vi "UI.vi"(0 "reference in":refnum<class "GUI Data Viewer.lvclass">, 5 "error in (no error)":errorcluster) -> (14 "reference out":refnum<class "GUI Data Viewer.lvclass">, 19 "error out":errorcluster)   [LabVIEW 2019, in "GUI Data Viewer.lvclass"]
uses:
  GUI Data Viewer.lvclass
  D:/GIT H4000/H4000/src/GUI_class/GUI.lvclass
  TypeDef/GUI Data Motor.ctl
  TypeDef/State Engine.ctl
  TypeDef/Needle Valve State.ctl
  GUI_class/GUI.lvclass/GUI.ctl
  TypeDef/AI_Data_Array.ctl
  TypeDef/AI_Data.ctl
  TypeDef/AI Statistics Data.ctl
  TypeDef/CalibrationData.ctl
  TypeDef/GUI Setting Channel.ctl
  TypeDef/GUI AI Ranges.ctl
  TypeDef/Scale Data.ctl
  SV_Wrap/SharedVariableWrapper.lvclass/SharedVariableWrapper.ctl
  TypeDef/Data Stand.ctl
  TypeDef/Mode.ctl
  TypeDef/ExecuteStepState.ctl
  TypeDef/Direction.ctl
  Modbus_class/STS REG.ctl
  TypeDef/SP_TYPE.ctl
  TypeDef/State 44-1-2.ctl
  Logger_class/Current Alarms.ctl
  Logger_class/EventData.ctl
  TypeDef/AlarmType.ctl
  TypeDef/error.ctl
  TypeDef/TCP Connection List.ctl
  <vilib>/NI/Modbus Library/Network Protocol/Network Slave/TCP/Connection.ctl
  TypeDef/Needle Valve Data.ctl
  modbus engine custom/MB_ENGINE_class/Engine State.ctl
  modbus engine custom/MB_ENGINE_class/Engine Alarms.ctl
  modbus engine custom/MB_ENGINE_class/Settings.ctl
  modbus engine custom/MB_ENGINE_class/Limits Status.ctl
  TypeDef/State PMG.ctl
  TypeDef/PMG Mode.ctl
  TypeDef/State Engine 2.ctl
  Modbus_class/CMD REG.ctl
  MessageAMC_class/MessageAMC.lvclass
  D:/GIT H4000/H4000/src/MessageInterface_class/MessageInterface.lvclass
  dd5645e7-7e6e-4691-95a0-f3999e380403.vi
  7c45c07e-402c-4694-b421-37bbb0792970.vi
  9a17e93e-f953-4ee5-a306-57728009cce8.vi
  49e40455-3b35-4e41-8043-7be2530b05e7.vi
  18541d12-0d59-4aa6-b87b-abaa8bd8a6e4.vi
  0b4675b1-6847-4ac1-af90-c3adb7e73b02.vi
  a37d2d01-2c81-48ed-b054-fbf1630c5e7f.vi
  1656e42f-8660-4372-8b8f-7d4878a983bb.vi
  0bfe0e00-7643-4872-b052-8b7f26ea950b.vi
  ffb61635-9317-4c26-9d6e-9a19723cfb80.vi
  07359d59-ff70-46be-ab7b-6b377f7d411b.vi
  f6869450-7c10-4810-a35a-46c2f9ab3114.vi
  d18fabfa-1a79-49d4-a75c-348c28269d79.vi
  d5087eaa-c132-4133-aa21-01cfea8cde9e.vi
  bf1f9f25-528c-4176-8d10-e7cb21e5fec2.vi
  e75bdee8-ee2a-4a87-80aa-f3e942366e41.vi
  f0a45f4a-50aa-43d2-a935-47ced4280b1d.vi
  cedc6c5e-9abe-42eb-b0bd-72af6e3c241b.vi
  GUI_class/Set Win State.vi
  GUI_class/protected/GetSheredData.vi
  dd5645e7-7e6e-4691-95a0-f3999e380403.vi/b5fe87cb-a842-48a6-ac33-23eb568e7aa4.vi
  SV_Wrap/Write Var Info.vi
  SV_Wrap/Read Var Info.vi
  7c45c07e-402c-4694-b421-37bbb0792970.vi/dcc16439-89b0-4283-9d30-44b050a4d697.vi
  49e40455-3b35-4e41-8043-7be2530b05e7.vi/daf86f20-c8fb-4d87-9d07-c45676e1c3eb.vi
  0b4675b1-6847-4ac1-af90-c3adb7e73b02.vi/1200fe38-aa22-4cab-916d-93cea7720ab1.vi
  a37d2d01-2c81-48ed-b054-fbf1630c5e7f.vi/408f54e3-e009-4e36-949a-cd8d2e669441.vi
  1656e42f-8660-4372-8b8f-7d4878a983bb.vi/3922be2e-8b70-4363-9278-b2eb396c106a.vi
  0bfe0e00-7643-4872-b052-8b7f26ea950b.vi/6182aae4-c240-425b-9f2c-7ffeca9a8282.vi
  07359d59-ff70-46be-ab7b-6b377f7d411b.vi/4407c637-9fa4-4312-8a7e-15880992c60d.vi
  f6869450-7c10-4810-a35a-46c2f9ab3114.vi/792ba656-e40c-479d-9018-d5581bd1c278.vi
  d18fabfa-1a79-49d4-a75c-348c28269d79.vi/30a4da04-0b22-486b-9a8e-f683f1398578.vi
  bf1f9f25-528c-4176-8d10-e7cb21e5fec2.vi/3b2418f1-7f16-47c7-ba27-2bc06ef6e628.vi
  e75bdee8-ee2a-4a87-80aa-f3e942366e41.vi/2202224e-9635-4547-b368-63a478ce0b2e.vi
  f0a45f4a-50aa-43d2-a935-47ced4280b1d.vi/85cd7a43-9f39-4f72-add9-b75505d0e5f9.vi
  cedc6c5e-9abe-42eb-b0bd-72af6e3c241b.vi/f9761a82-5467-46da-8b92-b56c6279bfed.vi
  SV_Wrap/Read connection str.vi
  <userlib>/_OpenG.lib/time/time.llb/Tick Count (ms)__ogtk.vi
  GUI_class/GUI.lvclass
  MessageInterface_class/MessageInterface.lvclass
  SV_Wrap/SharedVariableWrapper.lvclass
  modbus engine custom/MB_ENGINE_class/MB_ENGINE.lvclass
  <vilib>/NI/Modbus Library/Network Protocol/Network Slave/TCP/TCP Slave.lvclass
panel:
  out "chmbr 2":dbl(graph) caption="41.3 [МПа]"
  out "leak":dbl caption="Утечки [МПа/мин]" format="%.2f"
  out "modbus":bool caption="Модбас"
  out "size(s) 2":i32 caption="Кол-во активных"
  out "size(s)":i32 caption="Общее кол-во"
  out "Active":string[](array[string]) caption="Активные подключения"
  out "База данных":bool
  out "warning":bool caption="Предупреждение"
  out "alarm":bool caption="Авария"
  out "String":string
  in  "Tab Control":enum32{"Аварии / предупреждения", "Графики"}(tab)
  out "Multicolumn Listbox":i32(listbox)=-1
  in  "Clear Error":bool
  out "dut":T1(graph) caption="Образец [МПа]"
  out "chmbr":T1(graph) caption="Камера [МПа]"
  in  "remote":bool caption="Разрешить внешнее управление"
  out "P_DUT_MB":dbl caption="Образец  [МПа]" format="%.2f"
  out "P_CHMBR_MB":dbl caption="Камера [МПа]" format="%.2f"
  out "Angle 37 2":dbl caption="Угол, град" format="%#.1f град"
  out "StateValveModbus 2":T2
  out "StateValveModbus":T2
  in  "alarm press":bool
  out "Angle 37 1":dbl caption="Угол, град" format="%#.1f град"
  out "m24":T3
  out "m21":T3
  out "m12":T3
  out "AO 1":dbl caption="Напр. проп. клапан [В]" format="%.2f"
  out "AO 0":dbl caption="Напр.\nпроп.\nклапан [В]" format="%.2f"
  out "30":dbl(slide)=60.30534351145039 caption="НВД" scale=0.0..10.0
  in  "stop":bool
  out "Connect":bool caption="Подключение \nконтроллер"
  out "DO 7":bool caption="33.9"
  out "DO 6":bool caption="33.8"
  out "DO 11":bool caption="33.13"
  out "DO 8":bool caption="33.12"
  out "5.1":dbl(slide)=60.30534351145039 scale=0.0..100.0
  out "4.1":dbl(slide)=53.84615384615385 scale=0.0..100.0
  out "5.2":dbl(slide)=60.30534351145039 scale=0.0..100.0
  out "4.2":dbl(slide)=53.84615384615385 scale=0.0..100.0
  out "41.2 [МПа]":dbl(knob) scale=0.0..10.0
  out "41.1 [МПа]":dbl(knob) scale=0.0..10.0
  out "38.3 [МПа]":dbl(knob) scale=0.0..10.0
  out "38.2 [МПа]":dbl(knob) scale=0.0..10.0
  out "41.3 [МПа]":dbl(knob) scale=0.0..10.0
  out "38.1 [МПа]":dbl(knob) scale=0.0..500.0
  out "DO 18":bool caption="ВОЗДУХ"
  out "44.1":bool
  out "44.2":bool
  out "37.2":bool
  out "37.1":bool
  out "DO 14":bool caption="33.6"
  out "DO 16":bool caption="33.4"
  out "DO 15":bool caption="33.5"
  out "DO 13":bool caption="33.10"
  out "DO 12":bool caption="33.11"
  out "DO 17":bool caption="33.3"
  out "DO 10":bool caption="33.2"
  out "DO 9":bool caption="33.1"
  out "DO 5":bool caption="33.7"
  out "nitro":bool
  # "42  бюретка"
  # "Подключения модбас"
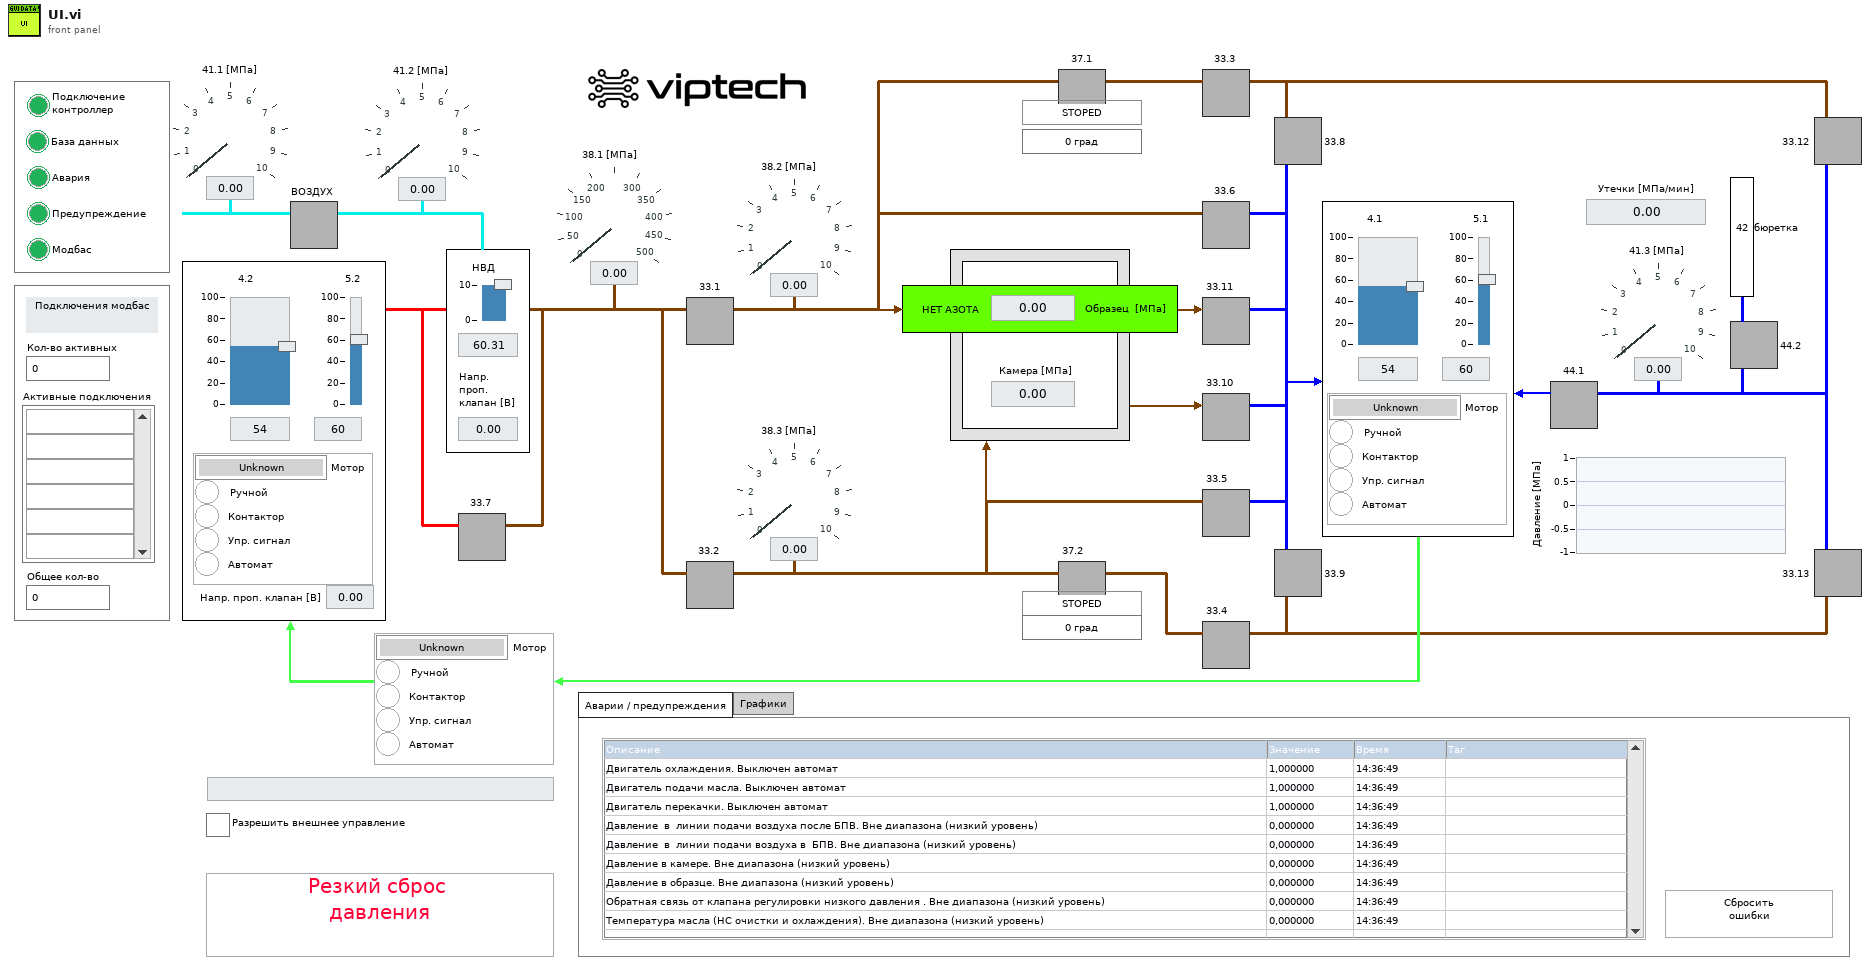
[diagram p1: front panel]
types:
  T1 = cluster{"Pressure SP":dbl, "scl mean 1Hz":dbl, "scl mean 1Hz":dbl}
  T2 = typedef "Needle Valve State.ctl" = enum16{"STOPED", "CLOSED", "OPENED", "OPENING", "CLOSING", "FULL_CLOSE"}
  T3 = typedef "GUI Data Motor.ctl" = cluster{"EngState":T4, "Active":bool, "Contactor":bool, "CMD":bool, "Automat":bool}
  T4 = typedef "State Engine.ctl" = enum16{"Unknown", "Off", "TupningOn", "On", "TurningOff"}
  T5 = typedef "CalibrationData.ctl" = cluster{"Channels":T6[], "Scales":T8[]}
  T6 = typedef "GUI Setting Channel.ctl" = cluster{"Name":string, "AI Ranges":T7, "ScaleIndex":u32}
  T7 = typedef "GUI AI Ranges.ctl" = cluster{"HI":bool, "HIHI":bool, "LO":bool, "LOLO":bool, "HIHI VAL":dbl, "HI VAL":dbl, "LO VAL":dbl, "LOLO VAL":dbl, "MAX RAW":dbl, "MIN RAW":dbl, "MAX SCALED":dbl, "MIN SCALED":dbl}
  T8 = typedef "Scale Data.ctl" = cluster{"index":i32, "Name":string, "X":dbl[], "Y":dbl[]}
  T9 = typedef "AI_Data_Array.ctl" = T10[]
  T10 = typedef "AI_Data.ctl" = cluster{"Stat Data":T11, "OutOfRangeMax":bool, "OutOfRangeMin":bool, "HIHI":bool, "HI":bool, "LO":bool, "LOLO":bool}
  T11 = typedef "AI Statistics Data.ctl" = cluster{"raw mean":dbl, "scl mean":dbl, "raw mean 1Hz":dbl, "scl mean 1Hz":dbl}
  T12 = typedef "Data Stand.ctl" = cluster{"CommCounter":u64, "BeginFilingLevel":dbl, "SP DUT":dbl, "SP CHAMBER":dbl, "Mode":T13, "ExecuteStepState":T14, "Direction":T15, "Direction Filling":T15, "mesuare start pressure [MPa]":dbl, "mesuare start time [s]":dbl, "mesuare velosity [MPA/s]":dbl, "STS":T16, "SP_TYPE_DUT":T17, "SP_TYPE_CHAMBER":T17, "New Step":bool, "BURETE_TIME":u16, "mesuare delta pressure [MPa]":dbl, "mesuare time [s]":dbl, "With BURETE":bool, "With Nitro":bool, "State 44-1-2":T18}
  T13 = typedef "Mode.ctl" = enum16{"IDLE", "FILLING", "EXECUTE_SP", "DRAIN"}
  T14 = typedef "ExecuteStepState.ctl" = enum16{"Init", "Set: Backpressure ", "Preload: HI", "Set: HI", "Maintenance: HI", "Down: Pressure"}
  T15 = typedef "Direction.ctl" = enum8{"DUT", "Chamber"}
  T16 = typedef "STS REG.ctl" = cluster{"IDLE":bool, "RYADY":bool, "STEP":bool, "ALARM":bool, "WARNING":bool, "REMOTE":bool, "SP_EXEC_DONE_DUT":bool, "SP_EXEC_DONE_CHAMBER":bool, "FILING_DONE_DUT":bool, "FILING_DONE_CHAMBER":bool, "BURETE_STATE":bool}
  T17 = typedef "SP_TYPE.ctl" = enum16{"ERROR", "ZIRO", "BASE", "SP"}
  T18 = typedef "State 44-1-2.ctl" = enum16{"Init", "Idle", "Wait", "Open 44-1", "Open 44-2", "Close 44-1", "Close 44-2"}
  T19 = typedef "Current Alarms.ctl" = cluster{"alarms":T20[]}
  T20 = typedef "EventData.ctl" = cluster{"obj_tag":string, "event_tag":string, "Description":string, "ALARM TYPE":T21, "Value DBL":dbl, "Value INT":i32, "Value STR":string, "Time Stamp":timestamp}
  T21 = typedef "AlarmType.ctl" = enum16{"Normal", "Warning", "Alarm"}
  T22 = typedef "error.ctl" = errorcluster
  T23 = typedef "TCP Connection List.ctl" = T24[]
  T24 = typedef "TCP Slave.lvclass/Connection.ctl" = cluster{"Connected?":bool, "IP address":string, "connection error":errorcluster}
  T25 = typedef "Needle Valve Data.ctl" = cluster{"Engine State":T26, "StateValveModbus":T2, "Alarms":T27, "RAW":i32, "Angele":dbl, "Step":i32, "Encoder":i32, "Kinematic":T28, "Limits":T29, "EncoderMax":i32, "Counter Max Dont Update":i32, "EncoderMin":i32, "Counter Min Dont Update":i32, "Prepere Counter":i32, "STEP INIT":i32, "offset - Angel":dbl}
  T26 = typedef "MB_ENGINE.lvclass/Engine State.ctl" = u16
  T27 = typedef "MB_ENGINE.lvclass/Engine Alarms.ctl" = cluster{"OL":bool, "TF":bool, "STL":bool, "OCP":bool, "CPUV":bool, "UVLO":bool, "SPI_ERROR":bool, "Fault":bool, "OL 2":bool, "TF 2":bool, "STL 2":bool, "OCP 2":bool, "CPUV 2":bool, "UVLO 2":bool, "reserved":bool, "InitDone":bool}
  T28 = typedef "MB_ENGINE.lvclass/Settings.ctl" = cluster{"ACC Steps Per Sec^2":u16, "DEC Steps Per Sec^2":u16, "Min Velosity Step Per Sec":u16, "Max Velosity Step Per Sec":u16, "MicroStep":u16}
  T29 = typedef "MB_ENGINE.lvclass/Limits Status.ctl" = cluster{"Fault 2 Switch":bool, "Fault 1 Switch":bool, "Center(Home)":bool, "Lower Limit":bool, "Upper Limit":bool}
  T30 = typedef "State PMG.ctl" = cluster{"PMG Mode":T31, "M12":T32, "M21":T32, "M24":T32}
  T31 = typedef "PMG Mode.ctl" = enum16{"Idel", "Filling", "Pressure"}
  T32 = typedef "State Engine 2.ctl" = cluster{"EngState":T4, "Active":bool, "Contactor":bool, "CMD":bool, "Automat":bool}
  T33 = cluster{"SP DUT":dbl, "scl mean 1Hz":dbl, "scl mean 1Hz":dbl}
  T34 = cluster{"SP CHAMBER":dbl, "scl mean 1Hz":dbl, "scl mean 1Hz":dbl}
  T35 = typedef "CMD REG.ctl" = cluster{"EXECUTE_SP":bool, "ALARM_PRESS_DOWN_DUT":bool, "ALARM_PRESS_DOWN_CHAMBER":bool, "ALARM_PRESS_DOWN_DUT_CHAMBER":bool, "FILING_DUT":bool, "FILING_CHAMBER":bool, "BLOCK":bool, "PUMP_STATION_OFF":bool, "OPEN_44_2":bool, "CLOSE_44_2":bool, "Drain":bool}
  T36 = enum32{"Invalid", "Standard", "Closed", "Hidden", "Minimized", "Maximized"}
  T37 = enum32{"invalid app kind", "Development System", "Run Time System", "Student Edition", "Embedded LabVIEW", "Evaluation", "Custom"}
  T38 = typedef "SharedVariableWrapper.lvclass/Config.ctl" = cluster{"connection str":string, "timeout":dbl, "ip":string}
  T39 = cluster{"Core":cluster{"Current VI Reference":refnum<vi>, "Close Panel on Exit?":bool}, "amc":refnum<class "MessageAMC.lvclass">}
  T40 = cluster{"Current VI Reference":refnum<vi>, "Close Panel on Exit?":bool}
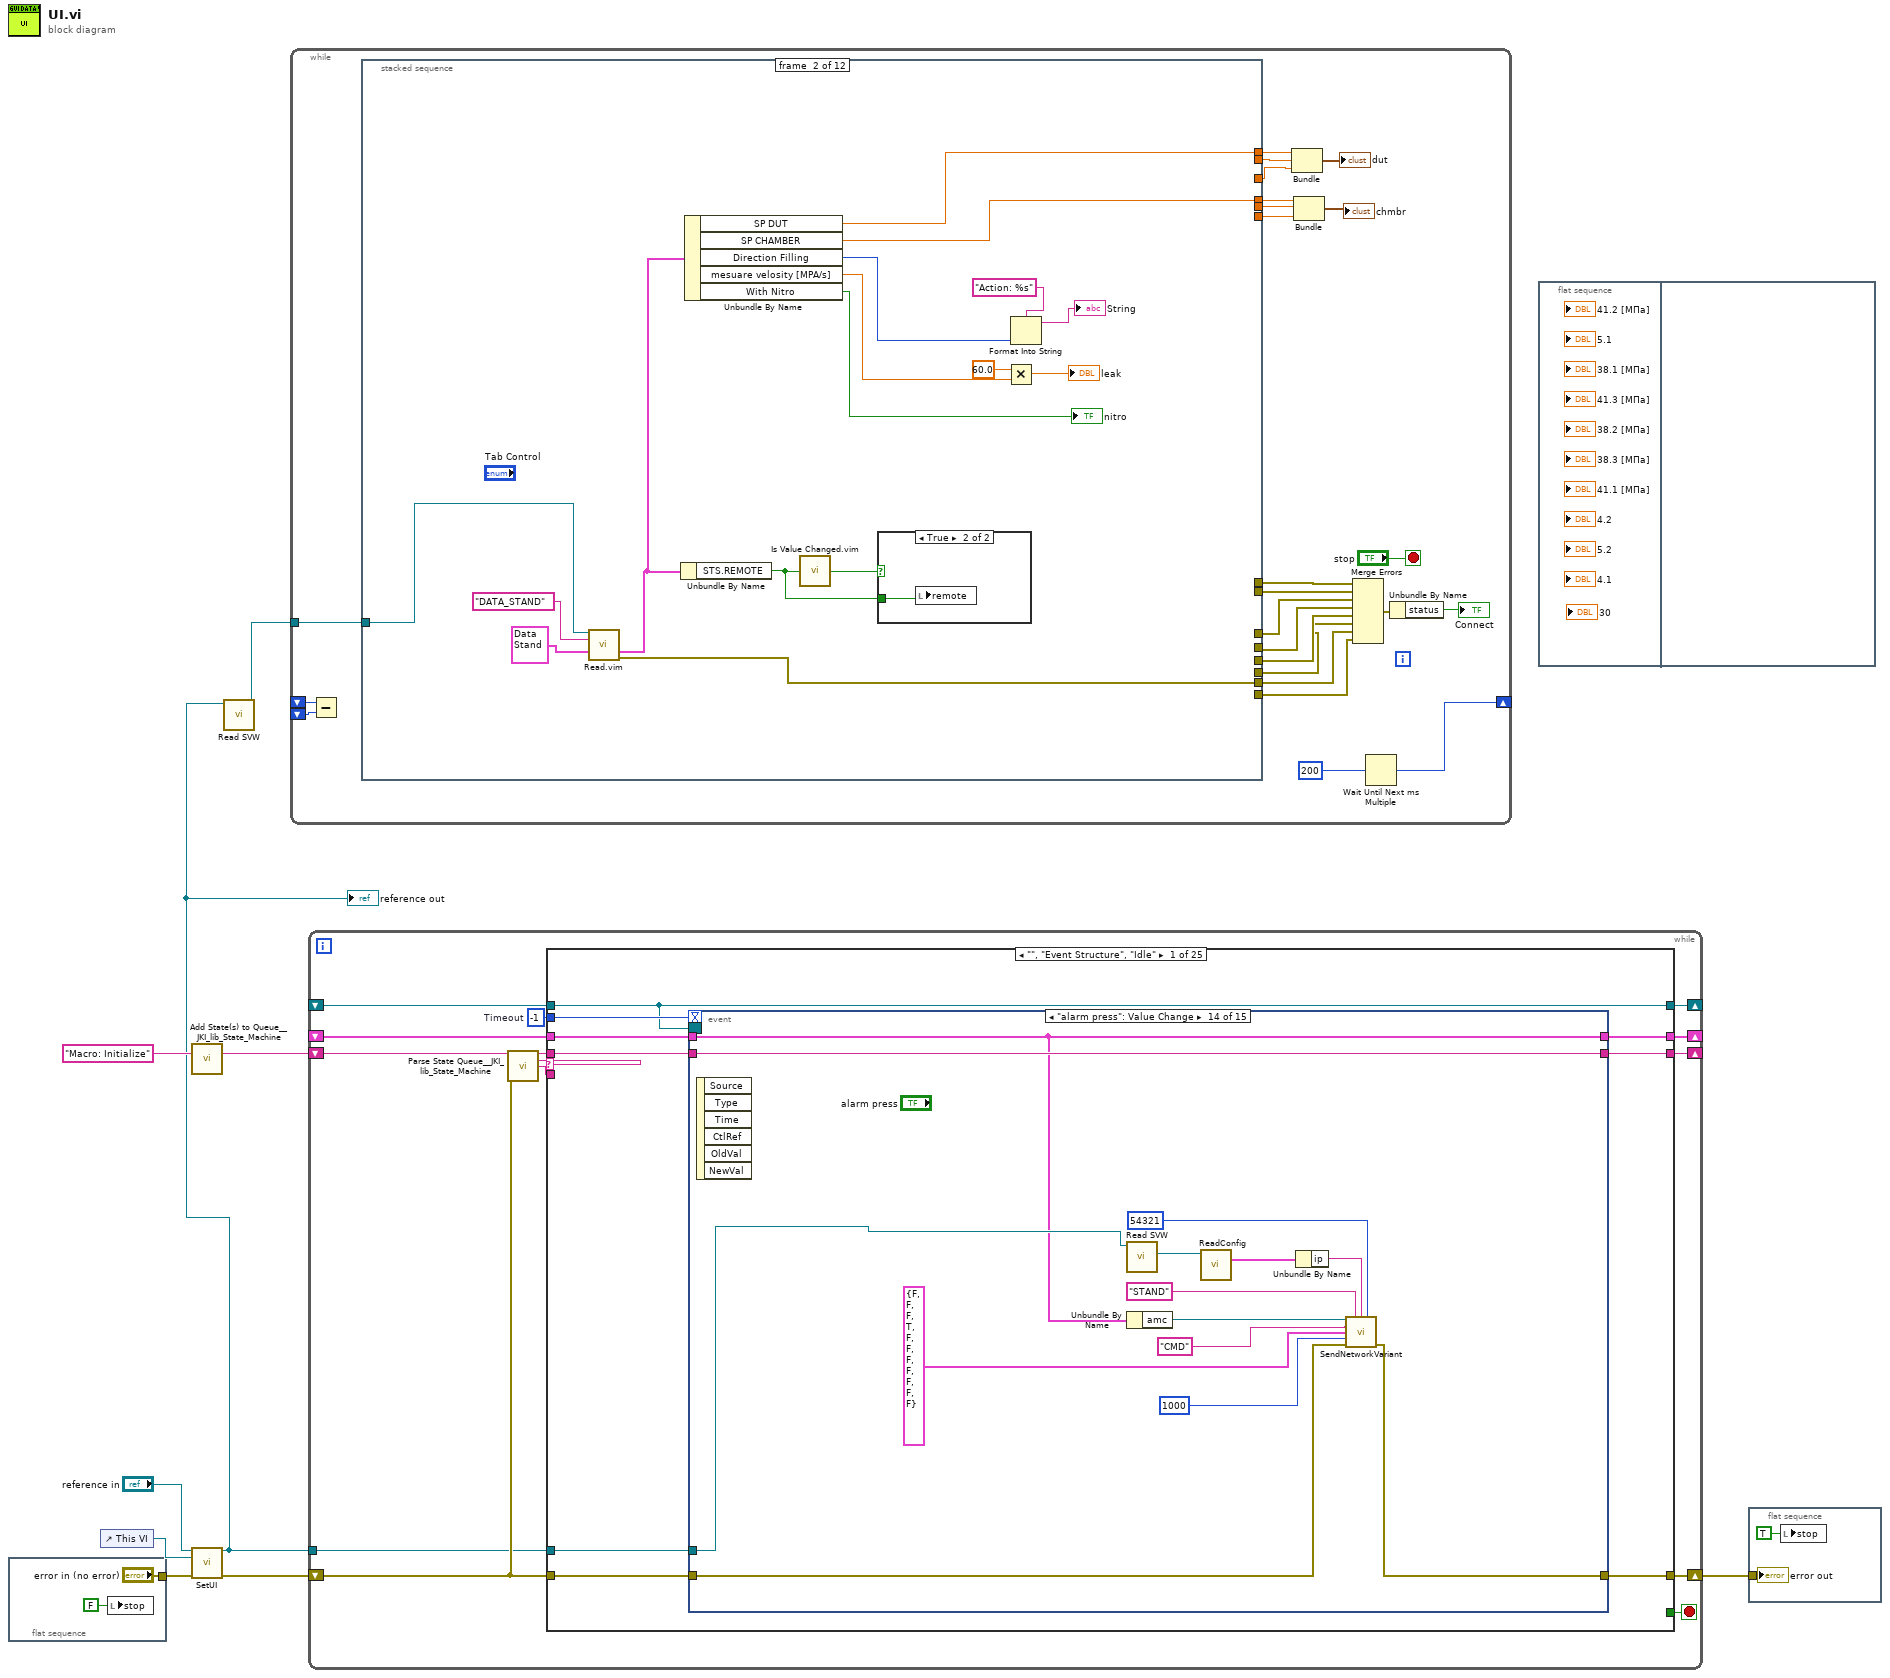
[diagram p0: block diagram]
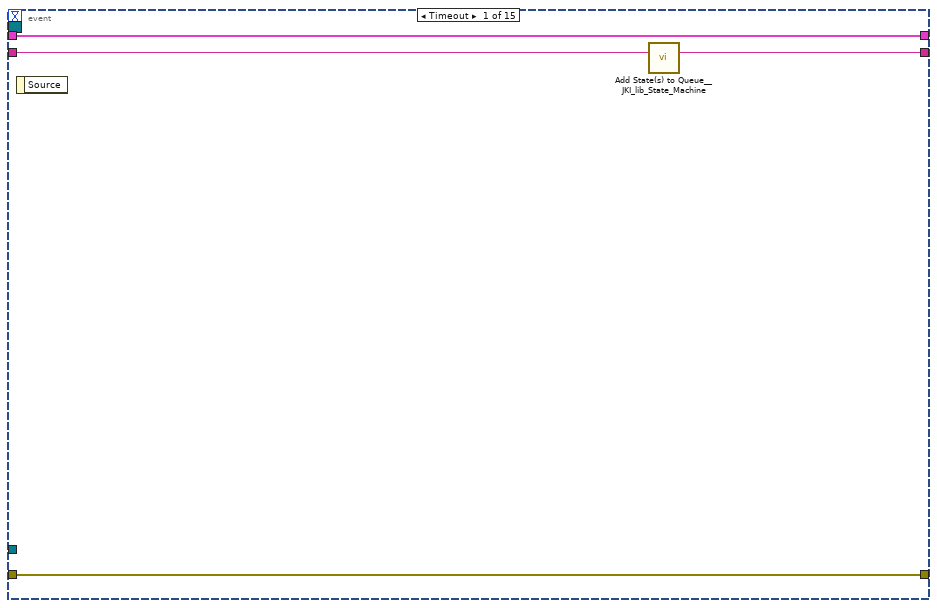
[diagram p2: hidden frame]
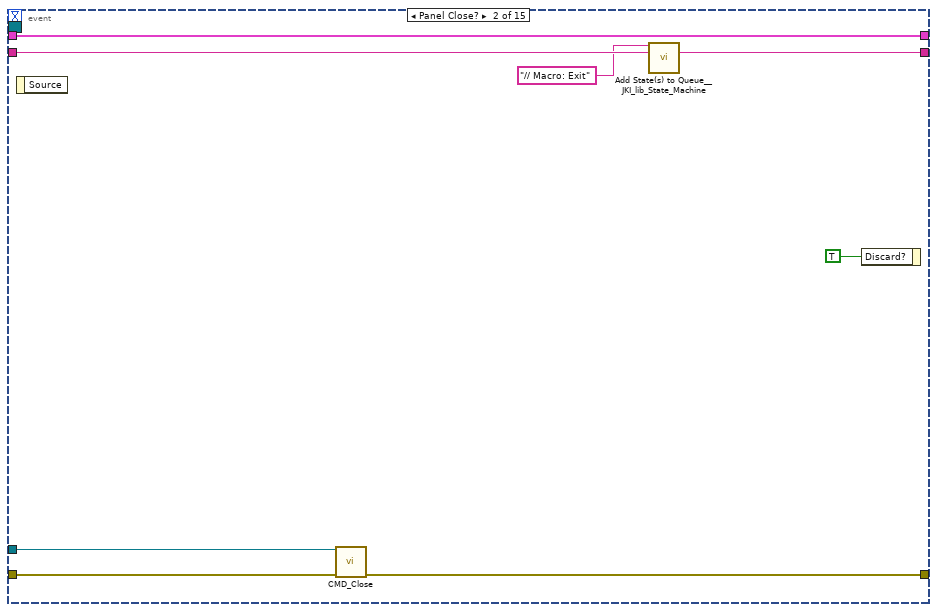
[diagram p3: hidden frame]
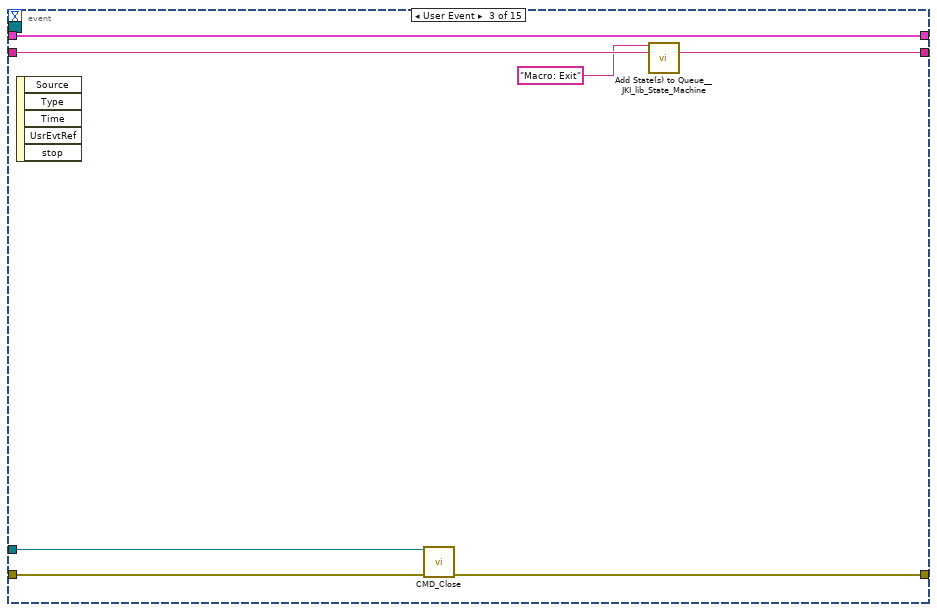
[diagram p4: hidden frame]
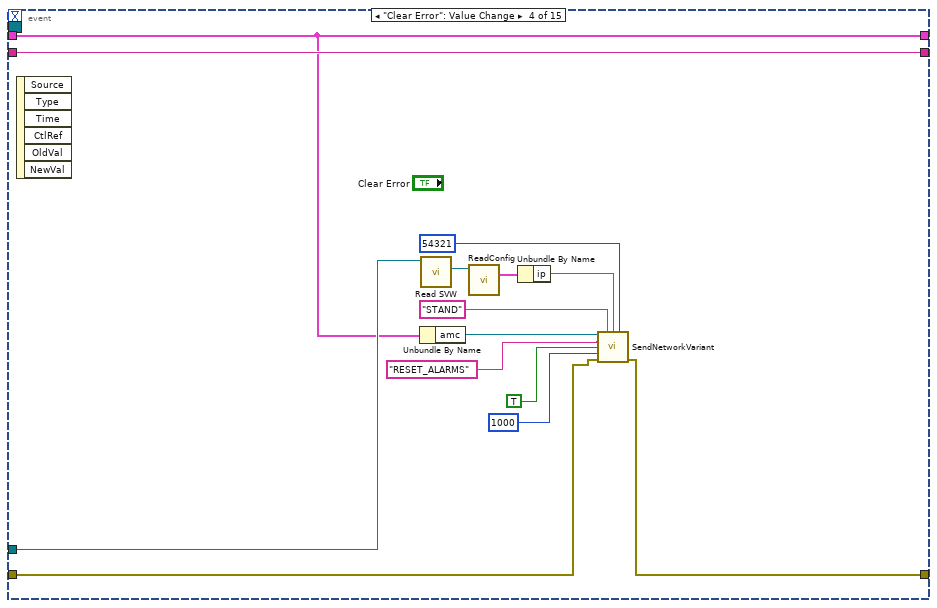
[diagram p5: hidden frame]
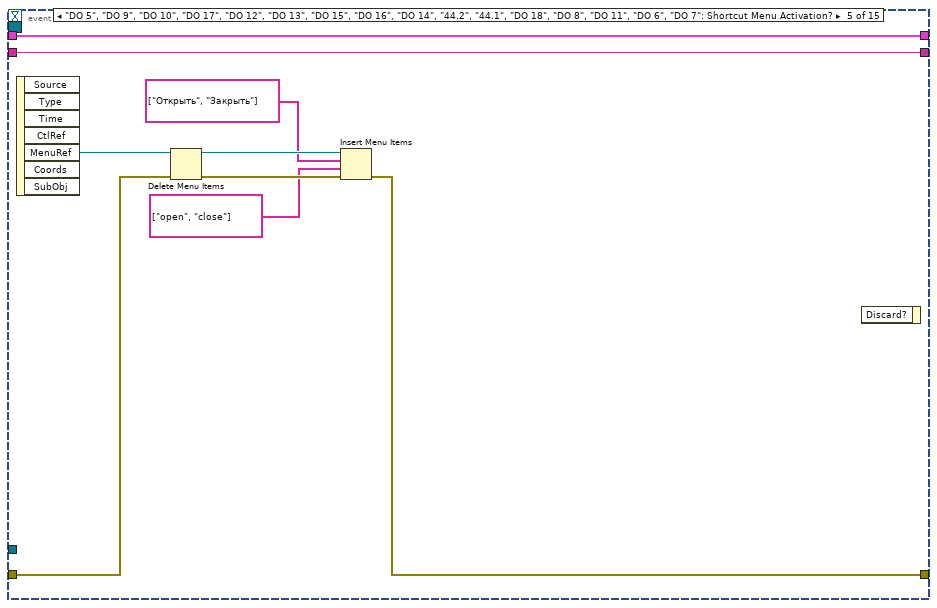
[diagram p6: hidden frame]
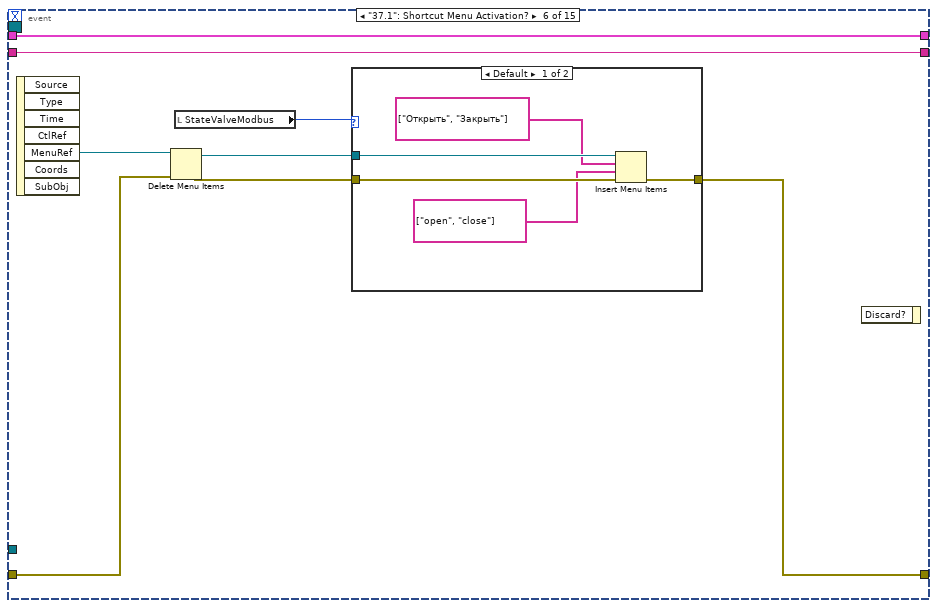
[diagram p7: hidden frame]
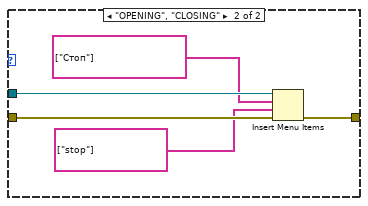
[diagram p8: hidden frame]
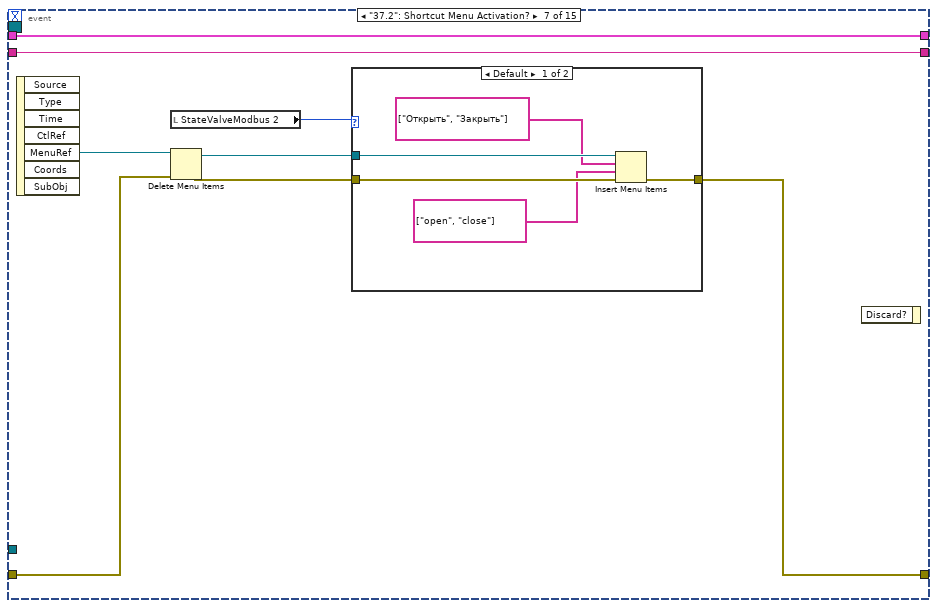
[diagram p9: hidden frame]
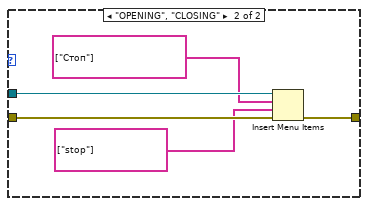
[diagram p10: hidden frame]
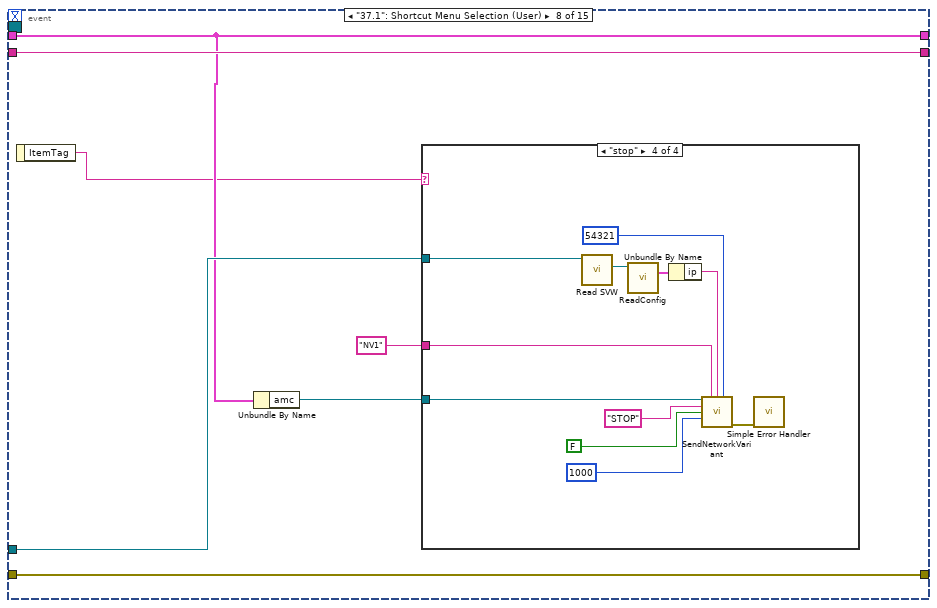
[diagram p11: hidden frame]
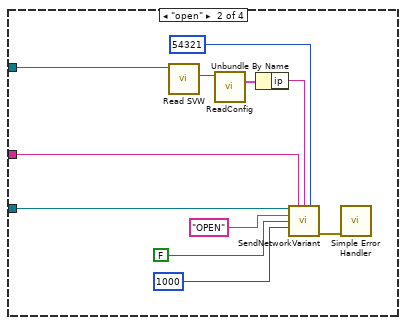
[diagram p13: hidden frame]
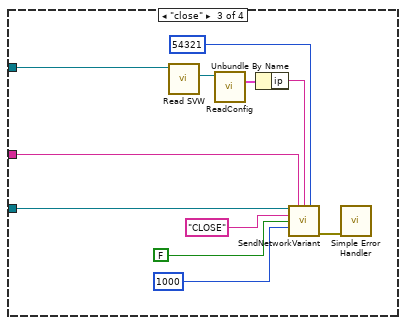
[diagram p14: hidden frame]
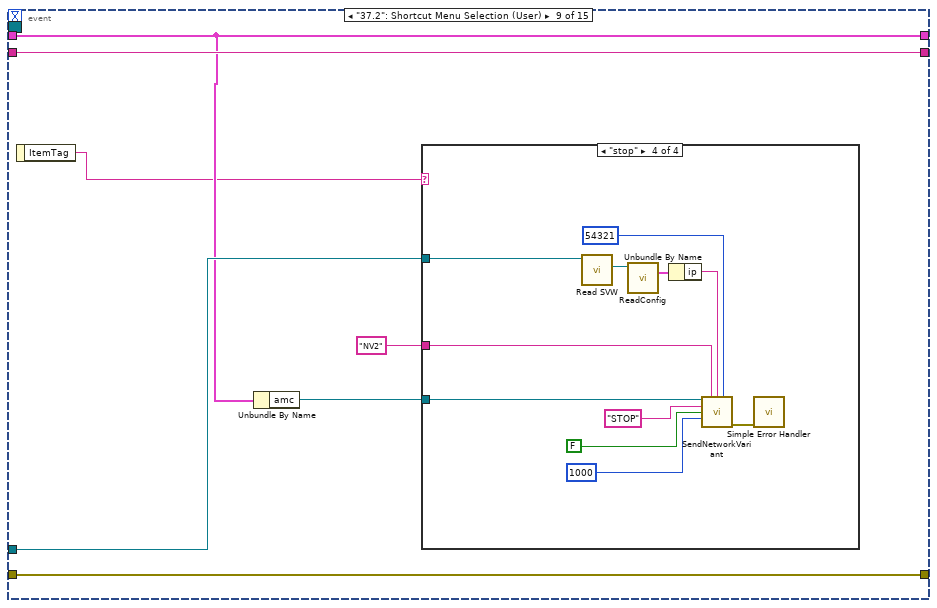
[diagram p15: hidden frame]
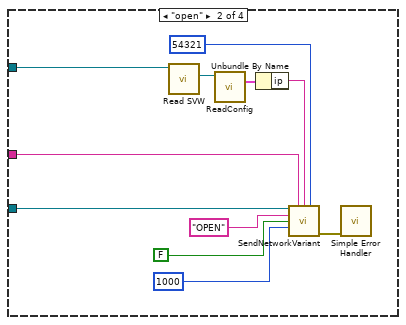
[diagram p17: hidden frame]
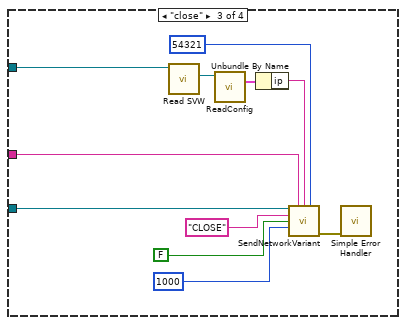
[diagram p18: hidden frame]
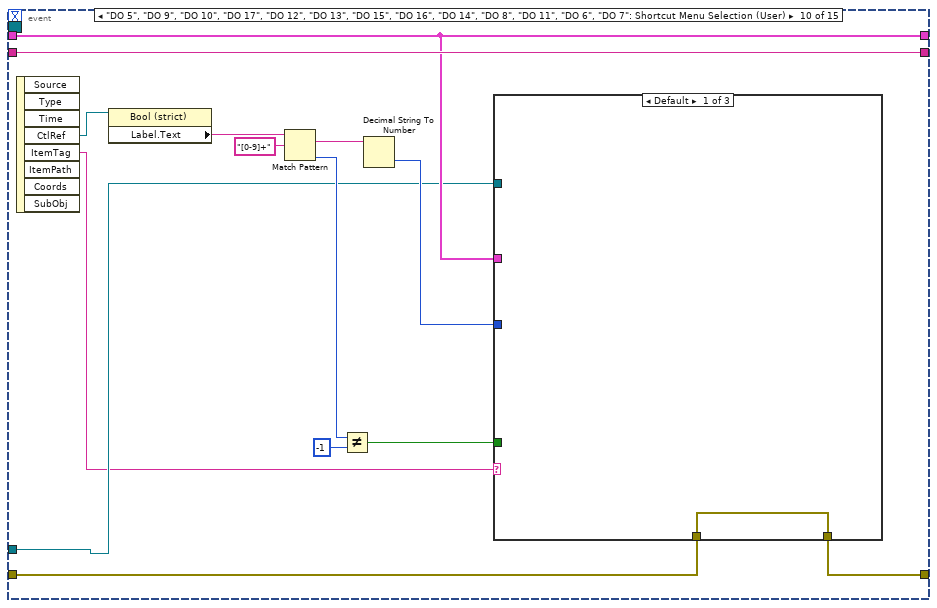
[diagram p19: hidden frame]
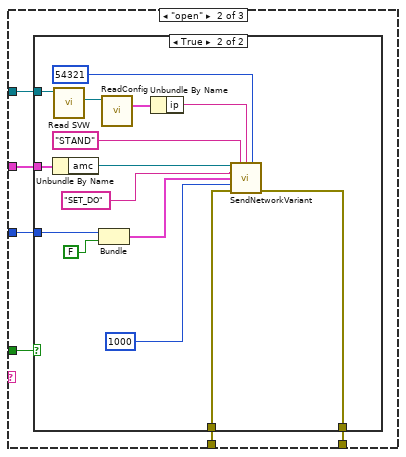
[diagram p20: hidden frame]
diagram:
  n1 = flat-sequence {
    tunnel: ["error in (no error)"] -> w6
    frame #0 {
      n2 = local write "stop"(FALSE ("stop")) -> ()
    }
  }
  n3 = control-ref of="This VI"() -> (w4:refnum<vi>)
  n4 = call <vilib>:"Add State(s) to Queue__JKI_lib_State_Machine.vi"("State(s) in (\"\")"="Macro: Initialize") -> ("States Out"=w9:string)  [unwired: 14 in]
  n5 = call "SetUI.vi"("reference in"="reference in", "UI VI"=w4, "error in (no error)"=w6) -> ("reference out"=w1:refnum<class "GUI Data Viewer.lvclass">, "error out"=w3:errorcluster)  [unwired: 11 in]
  "reference out" <- w1
  n6 = call "Read SVW.vi"("GUI in"=w1) -> ("SharedVariableWrapper.lvclass"=w2:refnum<class "SharedVariableWrapper.lvclass">)  [unwired: 10 in]
  n7 = while {
    tunnel: w2 -> [w33]
    shift-right: [w24] -> _
    shift-left: _ -> [w23]
    shift-left: _ -> [w22]
    stop <- "stop" stop-if-true
    n8 = Subtract(x=w23, y=w22) -> ()  [unwired: 1 out]
    n9 = stacked-sequence {
      tunnel: w33 -> [w70 w98 w106 w110 w126 w149 w159 w184 w210 w250 w251 w263]
      tunnel: [w72 _ _ _ _ _ _ _ _ _ _ _] -> w31
      tunnel: [_ _ _ _ _ _ _ _ w206 _ _ _] -> w32
      tunnel: [w71 _ _ _ _ _ _ _ _ _ _ _] -> w28
      tunnel: [_ _ w104 _ _ _ _ _ _ _ _ _] -> w27
      tunnel: [_ _ _ _ _ w146 _ _ _ _ _ _] -> w26
      tunnel: [_ _ _ _ _ _ _ w167 _ _ _ _] -> w25
      tunnel: [_ w97 _ _ _ _ _ _ _ _ _ _] -> w21
      tunnel: [_ w93 _ _ _ _ _ _ _ _ _ _] -> w18
      tunnel: [_ w92 _ _ _ _ _ _ _ _ _ _] -> w17
      tunnel: [_ _ _ _ _ _ w158 _ _ _ _ _] -> w16
      tunnel: [_ _ _ _ _ _ w157 _ _ _ _ _] -> w15
      tunnel: [w41 _ _ _ _ _ _ _ _ _ _ _] -> w14
      tunnel: [w39 _ _ _ _ _ _ _ _ _ _ _] -> w13
      tunnel: [_ _ _ _ w125 _ _ _ _ _ _ _] -> w12
      frame #0 {
        (unwired) T10 {"Stat Data"={"raw mean"=0.0, "scl mean"=0.0, "raw mean 1Hz"=0.0, "scl mean 1Hz"=0.0}, "OutOfRangeMax"=FALSE, "OutOfRangeMin"=FALSE, "HIHI"=FALSE, "HI"=FALSE, "LO"=FALSE, "LOLO"=FALSE} ("AI_Data")
        n10 = control-ref of="41.3 [МПа]"() -> (w57:refnum<vi>)
        n11 = control-ref of="38.1 [МПа]"() -> (w52:refnum<vi>)
        n12 = control-ref of="38.2 [МПа]"() -> (w53:refnum<vi>)
        n13 = control-ref of="38.3 [МПа]"() -> (w54:refnum<vi>)
        n14 = control-ref of="41.1 [МПа]"() -> (w55:refnum<vi>)
        n15 = control-ref of="41.2 [МПа]"() -> (w56:refnum<vi>)
        n16 = control-ref of="4.1"() -> (w46:refnum<vi>)
        n17 = control-ref of="5.1"() -> (w47:refnum<vi>)
        n18 = control-ref of="4.2"() -> (w48:refnum<vi>)
        n19 = control-ref of="5.2"() -> (w49:refnum<vi>)
        n20 = control-ref of="30"() -> (w50:refnum<vi>)
        n21 = Build Array(w52, w53, w54, w55, w56, w57) -> (w51:refnum<vi>[])
        n22 = Build Array(w46, w47, w48, w49, w50) -> (w45:refnum<vi>[])
        n23 = call "Read.vim"("SharedVariableWrapper in"=w70, "name"="AI_ARRAY", "DataType"=T9 [] ("AI_Data_Array")) -> ("connected"=w67:bool, "data out"=w44:T9, "error out"=w66:errorcluster)  [unwired: 6 in, 4 out]
        n24 = call "Read.vim"("SharedVariableWrapper in"=w70, "name"="CALIBRATION_DATA" ("VAR"), "DataType"=T5 {"Channels"=[], "Scales"=[]} ("CalibrationData")) -> ("data out"=w63:T5, "error out"=w61:errorcluster)  [unwired: 6 in, 5 out]
        n25 = Unbundle By Name(w63) -> ("Channels"=w62:T6[])
        n26 = Build Array (concatenate)(w45, w51) -> (w58:refnum<vi>[])
        n27 = Array Subset(array=w62, index=5) -> (w60:T6[])  [unwired: 1 in]
        n28 = Index Array(array=w44, index #1=6 ("index"), index #3=10 ("index")) -> (element #1=w42:T10, element #2=w40:T10, element #3=w37:T10)  [unwired: 1 in]
        n29 = for {
          tunnel: w67 -> [w81]
          tunnel: w44 -> [w82]
          shift-right: [w83] -> w72
          shift-left: w66 -> [w84]
          tunnel: w58 -> [w78] mode=indexing
          i -> [w79]
          n30 = Index Array(array=w82, index=w79) -> (element=w80:T10)
          n31 = call "UpdateNumericWithScale.vi"("NumericWithScale in"=w78, "connect"=w81, "AI_Data"=w80, "error in (no error)"=w84) -> ("error out"=w83:errorcluster)  [unwired: 11 in]
        }
        n32 = for {
          tunnel: w51 -> [w77] mode=indexing
          tunnel: w60 -> [w76] mode=indexing
          shift-right: [w74] -> w71
          shift-left: w61 -> [w73]
          n33 = Unbundle By Name(w76) -> ("AI Ranges"=w75:T7)
          n34 = call "Set Color Zones.vim"("reference"=w77, "AI Ranges"=w75, "error in (no error)"=w73) -> ("error out"=w74:errorcluster)  [unwired: 12 in]
        }
        n35 = Unbundle By Name(w42) -> ("Stat Data.scl mean 1Hz"=w41:dbl)
        n36 = Unbundle By Name(w37) -> ("Stat Data.scl mean 1Hz"=→"chmbr 2":dbl)
        n37 = Unbundle By Name(w40) -> ("Stat Data.scl mean 1Hz"=w39:dbl)
      }
      frame #1 {
        n38 = call "Read.vim"("SharedVariableWrapper in"=w98, "name"="DATA_STAND", "DataType"=T12 {"CommCounter"=0, "BeginFilingLevel"=0.0, "SP DUT"=0.0, "SP CHAMBER"=0.0, "Mode"=enum."IDLE", "ExecuteStepState"=enum."Init", "Direction"=enum."DUT", "Direction Filling"=enum."DUT", "mesuare start pressure [MPa]"=0.0, "mesuare start time [s]"=0.0, "mesuare velosity [MPA/s]"=0.0, "STS"={"IDLE"=FALSE, "RYADY"=FALSE, "STEP"=FALSE, "ALARM"=FALSE, "WARNING"=FALSE, "REMOTE"=FALSE, "SP_EXEC_DONE_DUT"=FALSE, "SP_EXEC_DONE_CHAMBER"=FALSE, "FILING_DONE_DUT"=FALSE, "FILING_DONE_CHAMBER"=FALSE, "BURETE_STATE"=FALSE}, "SP_TYPE_DUT"=enum."ZIRO", "SP_TYPE_CHAMBER"=enum."ZIRO", "New Step"=FALSE, "BURETE_TIME"=0, "mesuare delta pressure [MPa]"=0.0, "mesuare time [s]"=0.0, "With BURETE"=FALSE, "With Nitro"=FALSE, "State 44-1-2"=enum."Init"} ("Data Stand")) -> ("data out"=w94:T12, "error out"=w97:errorcluster)  [unwired: 6 in, 5 out]
        n39 = Unbundle By Name(w94) -> ("STS.REMOTE"=w96:bool)
        n40 = Unbundle By Name(w94) -> ("SP DUT"=w93:dbl, "SP CHAMBER"=w92:dbl, "Direction Filling"=w89:T15, "mesuare velosity [MPA/s]"=w88:dbl, "With Nitro"=→"nitro":bool)
        n41 = call "Is Value Changed.vim"("value"=w96) -> ("changed or first call?"=w95:bool)
        n42 = case shown="True" w95 {
          tunnel: w96 -> [_ w101]
          frame False {
          }
          frame True {
            n43 = local write "remote"(w101) -> ()
          }
        }
        n44 = Multiply(x=60.0, y=w88) -> (x*y=→"leak":dbl)
        n45 = Format Into String(format string="Action: %s", w89) -> (resulting string=→"String":string)  [unwired: 2 in, 1 out]
      }
      frame #2 {
        n46 = control-ref of="Multicolumn Listbox"() -> (w109:refnum<vi>)
        n47 = call "Read.vim"("SharedVariableWrapper in"=w106, "name"="CURRENT_ALARMS", "DataType"=T19 {"alarms"=[{"obj_tag"="AI0", "event_tag"="AI0.OUT_OF_RANGE_MIN", "Description"="Уровень  масла (НС очистки и охлаждения). Вне диапазона (низкий уровень)", "ALARM TYPE"=enum."Alarm", "Value DBL"=0.0, "Value INT"=1, "Value STR"="Alarm", "Time Stamp"=timestamp(3830845009.237916 s since 1904-01-01)}, {"obj_tag"="AI1", "event_tag"="AI1.OUT_OF_RANGE_MIN", "Description"="Уровень масла (НС подачи масла). Вне диапазона (низкий уровень)", "ALARM TYPE"=enum."Alarm", "Value DBL"=0.0, "Value INT"=1, "Value STR"="Alarm", "Time Stamp"=timestamp(3830845009.237916 s since 1904-01-01)}, {"obj_tag"="AI10", "event_tag"="AI10.OUT_OF_RANGE_MIN", "Description"="Датчик давления в линии измерения утечек. Вне диапазона (низкий уровень)", "ALARM TYPE"=enum."Alarm", "Value DBL"=0.0, "Value INT"=1, "Value STR"="Alarm", "Time Stamp"=timestamp(3830845009.237916 s since 1904-01-01)}, {"obj_tag"="AI2", "event_tag"="AI2.OUT_OF_RANGE_MIN", "Description"="Температура масла (НС очистки и охлаждения). Вне диапазона (низкий уровень)", "ALARM TYPE"=enum."Alarm", "Value DBL"=0.0, "Value INT"=1, "Value STR"="Alarm", "Time Stamp"=timestamp(3830845009.237916 s since 1904-01-01)}, {"obj_tag"="AI3", "event_tag"="AI3.OUT_OF_RANGE_MIN", "Description"="Температура масла (НС подачи масла). Вне диапазона (низкий уровень)", "ALARM TYPE"=enum."Alarm", "Value DBL"=0.0, "Value INT"=1, "Value STR"="Alarm", "Time Stamp"=timestamp(3830845009.237916 s since 1904-01-01)}, {"obj_tag"="AI4", "event_tag"="AI4.OUT_OF_RANGE_MIN", "Description"="Обратная связь от клапана регулировки низкого давления . Вне диапазона (низкий уровень)", "ALARM TYPE"=enum."Alarm", "Value DBL"=0.0, "Value INT"=1, "Value STR"="Alarm", "Time Stamp"=timestamp(3830845009.237916 s since 1904-01-01)}, {"obj_tag"="AI5", "event_tag"="AI5.OUT_OF_RANGE_MIN", "Description"="Давление после насоса ВД. Вне диапазона (низкий уровень)", "ALARM TYPE"=enum."Alarm", "Value DBL"=0.0, "Value INT"=1, "Value STR"="Alarm", "Time Stamp"=timestamp(3830845009.237916 s since 1904-01-01)}, {"obj_tag"="AI6", "event_tag"="AI6.OUT_OF_RANGE_MIN", "Description"="Давление в образце. Вне диапазона (низкий уровень)", "ALARM TYPE"=enum."Alarm", "Value DBL"=0.0, "Value INT"=1, "Value STR"="Alarm", "Time Stamp"=timestamp(3830845009.237916 s since 1904-01-01)}, {"obj_tag"="AI7", "event_tag"="AI7.OUT_OF_RANGE_MIN", "Description"="Давление в камере. Вне диапазона (низкий уровень)", "ALARM TYPE"=enum."Alarm", "Value DBL"=0.0, "Value INT"=1, "Value STR"="Alarm", "Time Stamp"=timestamp(3830845009.237916 s since 1904-01-01)}, {"obj_tag"="AI8", "event_tag"="AI8.OUT_OF_RANGE_MIN", "Description"="Давление  в  линии подачи воздуха в  БПВ. Вне диапазона (низкий уровень)", "ALARM TYPE"=enum."Alarm", "Value DBL"=0.0, "Value INT"=1, "Value STR"="Alarm", "Time Stamp"=timestamp(3830845009.237916 s since 1904-01-01)}, {"obj_tag"="AI9", "event_tag"="AI9.OUT_OF_RANGE_MIN", "Description"="Давление  в  линии подачи воздуха после БПВ. Вне диапазона (низкий уровень)", "ALARM TYPE"=enum."Alarm", "Value DBL"=0.0, "Value INT"=1, "Value STR"="Alarm", "Time Stamp"=timestamp(3830845009.237916 s since 1904-01-01)}, {"obj_tag"="M12", "event_tag"="M12.AUTOMAT_ERROR", "Description"="Двигатель перекачки. Выключен автомат", "ALARM TYPE"=enum."Alarm", "Value DBL"=1.0, "Value INT"=1, "Value STR"="Alarm", "Time Stamp"=timestamp(3830845009.739716 s since 1904-01-01)}, {"obj_tag"="M21", "event_tag"="M21.AUTOMAT_ERROR", "Description"="Двигатель подачи масла. Выключен автомат", "ALARM TYPE"=enum."Alarm", "Value DBL"=1.0, "Value INT"=1, "Value STR"="Alarm", "Time Stamp"=timestamp(3830845009.739716 s since 1904-01-01)}, {"obj_tag"="M22", "event_tag"="M22.AUTOMAT_ERROR", "Description"="Двигатель охлаждения. Выключен автомат", "ALARM TYPE"=enum."Alarm", "Value DBL"=1.0, "Value INT"=1, "Value STR"="Alarm", "Time Stamp"=timestamp(3830845009.739716 s since 1904-01-01)}]} ("data in")) -> ("data out"=w105:T19, "error out"=w104:errorcluster)  [unwired: 6 in, 5 out]
        n48 = call "GUI Alarms Tbl.vi"("data in"=w105, "Multicolumn Listbox ref"=w109) -> ("alarms"=→"alarm":bool, "warning"=→"warning":bool)  [unwired: 12 in]
      }
      frame #3 {
        n49 = call "Read.vim"("SharedVariableWrapper in"=w110, "name"="ERROR_BD", "DataType"=T22 {"status"=FALSE, "code"=0, "source"=""} ("error")) -> ("data out"=w112:T22, "error out"=w114:errorcluster)  [unwired: 6 in, 5 out]
        n50 = Unbundle By Name(w112) -> ("status"=→"База данных":bool)
        n51 = call <vilib>:"Clear Errors.vi"("error in (no error)"=w114) -> ()  [unwired: 5 in, 2 out]
      }
      frame #4 {
        n52 = call "Read.vim"("SharedVariableWrapper in"=w126, "name"="TCP_Connection_List", "DataType"=T23 [] ("TCP Connection List")) -> ("data out"=w123:T23, "error out"=w125:errorcluster)  [unwired: 6 in, 5 out]
        n53 = for {
          tunnel: w123 -> [w130] mode=indexing
          tunnel: [w129] -> w120 mode=indexing if=w128
          n54 = Unbundle By Name(w130) -> ("IP address"=w129:string, "Connected?"=w128:bool)
        }
        "Active" <- w120
        n55 = Array Size(array=w123) -> (size(s)=→"size(s)":i32)
        n56 = Array Size(array=w120) -> (size(s)=→"size(s) 2":i32)
        n57 = Search 1D Array(1D array=w120, element="192.168.2.10") -> (index of element=w118:i32)  [unwired: 1 in]
        n58 = Equal?(x=w118, y=-1) -> (x = y?=→"modbus":bool)
      }
      frame #5 {
        n59 = call "Read.vim"("SharedVariableWrapper in"=w149, "name"="NV1_DATA", "DataType"=T25 {"Engine State"=8, "StateValveModbus"=enum."STOPED", "Alarms"={"OL"=FALSE, "TF"=FALSE, "STL"=FALSE, "OCP"=FALSE, "CPUV"=FALSE, "UVLO"=FALSE, "SPI_ERROR"=FALSE, "Fault"=FALSE, "OL 2"=FALSE, "TF 2"=FALSE, "STL 2"=FALSE, "OCP 2"=FALSE, "CPUV 2"=FALSE, "UVLO 2"=FALSE, "reserved"=TRUE, "InitDone"=TRUE}, "RAW"=124110, "Angele"=0.0, "Step"=0, "Encoder"=0, "Kinematic"={"ACC Steps Per Sec^2"=100, "DEC Steps Per Sec^2"=100, "Min Velosity Step Per Sec"=100, "Max Velosity Step Per Sec"=200, "MicroStep"=16}, "Limits"={"Fault 2 Switch"=FALSE, "Fault 1 Switch"=FALSE, "Center(Home)"=FALSE, "Lower Limit"=FALSE, "Upper Limit"=FALSE}, "EncoderMax"=0, "Counter Max Dont Update"=0, "EncoderMin"=0, "Counter Min Dont Update"=0, "Prepere Counter"=0, "STEP INIT"=0, "offset - Angel"=0.0} ("NVM Data")) -> ("data out"=w150:T25, "error out"=w146:errorcluster)  [unwired: 6 in, 5 out]
        n60 = Unbundle By Name(w150) -> ("Alarms"=w145:T27, "StateValveModbus"=w133:T2, "offset - Angel"=→"Angle 37 1":dbl)  [unwired: 2 out]
        "StateValveModbus" <- w133
        n61 = Unbundle By Name(w145) -> ("OL"=w144:bool, "TF"=w143:bool, "STL"=w142:bool, "OCP"=w141:bool, "CPUV"=w140:bool, "UVLO"=w139:bool, "SPI_ERROR"=w138:bool, "Fault"=w137:bool, "InitDone"=w136:bool)
        n62 = feedback #1() -> (w132:bool)  [unwired: 1 in]
        n63 = case shown="\"STOPED\", \"OPENED\"" w133 {
          tunnel: [w152 FALSE TRUE] -> w131
          tunnel: w132 -> [w153 _ _]
          frame Default {
            n64 = Not(x=w153) -> (.not. x?=w152:bool)
          }
          frame "CLOSED" {
          }
          frame "STOPED", "OPENED" {
          }
        }
        "37.1" <- w131
        n65 = feedback-in #1(w131) -> ()
        n66 = Compound Arithmetic op=OR(w144, w143, w142, w141, w140, w139, w138, w137, invert w136) -> (w135:bool)
        n67 = call "Is Value Changed.vim"("value"=w135) -> ("changed or first call?"=w134:bool)
        n68 = case shown="True" w134 {
          tunnel: w135 -> [_ w156]
          frame False {
          }
          frame True {
            n69 = property on="37.1" class="Bool (strict)"("Blinking"=w156) -> ()  [unwired: 2 in, 2 out]
          }
        }
      }
      frame #6 {
        w162 = T10 {"Stat Data"={"raw mean"=0.0, "scl mean"=0.0, "raw mean 1Hz"=0.0, "scl mean 1Hz"=0.0}, "OutOfRangeMax"=FALSE, "OutOfRangeMin"=FALSE, "HIHI"=FALSE, "HI"=FALSE, "LO"=FALSE, "LOLO"=FALSE} ("AI_Data")
        n70 = call "Read.vim"("SharedVariableWrapper in"=w159, "name"="P_CHMBR_MB", "DataType"=w162) -> ("data out"=w160:T10, "error out"=w163:errorcluster)  [unwired: 6 in, 5 out]
        n71 = call "Read.vim"("SharedVariableWrapper in"=w159, "name"="P_DUT_MB", "DataType"=w162, "error in (no error)"=w163) -> ("data out"=w161:T10)  [unwired: 5 in, 6 out]
        n72 = Unbundle By Name(w160) -> ("Stat Data.scl mean 1Hz"=w157:dbl)
        "P_CHMBR_MB" <- w157
        n73 = Unbundle By Name(w161) -> ("Stat Data.scl mean 1Hz"=w158:dbl)
        "P_DUT_MB" <- w158
      }
      frame #7 {
        n74 = call "Read.vim"("SharedVariableWrapper in"=w184, "name"="NV2_DATA", "DataType"=T25 {"Engine State"=8, "StateValveModbus"=enum."STOPED", "Alarms"={"OL"=FALSE, "TF"=FALSE, "STL"=FALSE, "OCP"=FALSE, "CPUV"=FALSE, "UVLO"=FALSE, "SPI_ERROR"=FALSE, "Fault"=FALSE, "OL 2"=FALSE, "TF 2"=FALSE, "STL 2"=FALSE, "OCP 2"=FALSE, "CPUV 2"=FALSE, "UVLO 2"=FALSE, "reserved"=TRUE, "InitDone"=TRUE}, "RAW"=124110, "Angele"=0.0, "Step"=0, "Encoder"=0, "Kinematic"={"ACC Steps Per Sec^2"=100, "DEC Steps Per Sec^2"=100, "Min Velosity Step Per Sec"=100, "Max Velosity Step Per Sec"=200, "MicroStep"=16}, "Limits"={"Fault 2 Switch"=FALSE, "Fault 1 Switch"=FALSE, "Center(Home)"=FALSE, "Lower Limit"=FALSE, "Upper Limit"=FALSE}, "EncoderMax"=0, "Counter Max Dont Update"=0, "EncoderMin"=0, "Counter Min Dont Update"=0, "Prepere Counter"=0, "STEP INIT"=0, "offset - Angel"=0.0} ("NVM Data")) -> ("data out"=w185:T25, "error out"=w167:errorcluster)  [unwired: 6 in, 5 out]
        n75 = Unbundle By Name(w185) -> ("Alarms"=w181:T27, "StateValveModbus"=w169:T2, "offset - Angel"=→"Angle 37 2":dbl)  [unwired: 2 out]
        "StateValveModbus 2" <- w169
        n76 = Unbundle By Name(w181) -> ("OL"=w180:bool, "TF"=w179:bool, "STL"=w178:bool, "OCP"=w177:bool, "CPUV"=w176:bool, "UVLO"=w175:bool, "SPI_ERROR"=w174:bool, "Fault"=w173:bool, "InitDone"=w172:bool)
        n77 = feedback #2() -> (w168:bool)  [unwired: 1 in]
        n78 = case shown="\"STOPED\", \"OPENED\"" w169 {
          tunnel: [w187 FALSE TRUE] -> w166
          tunnel: w168 -> [w188 _ _]
          frame Default {
            n79 = Not(x=w188) -> (.not. x?=w187:bool)
          }
          frame "CLOSED" {
          }
          frame "STOPED", "OPENED" {
          }
        }
        "37.2" <- w166
        n80 = feedback-in #2(w166) -> ()
        n81 = Compound Arithmetic op=OR(w180, w179, w178, w177, w176, w175, w174, w173, invert w172) -> (w171:bool)
        n82 = call "Is Value Changed.vim"("value"=w171) -> ("changed or first call?"=w170:bool)
        n83 = case shown="True" w170 {
          tunnel: w171 -> [_ w191]
          frame False {
          }
          frame True {
            n84 = property on="37.2" class="Bool (strict)"("Blinking"=w191) -> ()  [unwired: 2 in, 2 out]
          }
        }
      }
      frame #8 {
        n85 = call "Read.vim"("SharedVariableWrapper in"=w210, "name"="DI_ARRAY", "DataType"=bool[] []) -> ("data out"=w207:bool[], "error out"=w206:errorcluster)  [unwired: 6 in, 5 out]
        n86 = Index Array(array=w207, index #1=21 ("index"), index #3=29 ("index")) -> (element #1=w203:bool, element #2=w202:bool, element #3=w201:bool, element #4=w200:bool)  [unwired: 2 in]
        n87 = Build Array(w203, w202) -> (w199:bool[])
        n88 = Build Array(w201, w200) -> (w198:bool[])
        n89 = Boolean Array To Number(Boolean array=w199) -> (number=w197:u32)
        n90 = Boolean Array To Number(Boolean array=w198) -> (number=w193:u32)
        n91 = feedback #3() -> (w194:bool)  [unwired: 1 in]
        n92 = case shown="1" w193 {
          tunnel: [w211 TRUE ("44.1") FALSE ("44.1")] -> w192
          tunnel: w194 -> [w212 _ _]
          frame Default {
            n93 = Not(x=w212) -> (.not. x?=w211:bool)
          }
          frame 1 {
          }
          frame 2 {
          }
        }
        "44.2" <- w192
        n94 = feedback-in #3(w192) -> ()
        n95 = feedback #4() -> (w195:bool)  [unwired: 1 in]
        n96 = case shown="Default" w197 {
          tunnel: [w215 TRUE ("44.1") FALSE ("44.1")] -> w196
          tunnel: w195 -> [w216 _ _]
          frame Default {
            n97 = Not(x=w216) -> (.not. x?=w215:bool)
          }
          frame 1 {
          }
          frame 2 {
          }
        }
        "44.1" <- w196
        n98 = feedback-in #4(w196) -> ()
      }
      frame #9 {
        n99 = call "Read.vim"("SharedVariableWrapper in"=w250, "name"="DO_ARRAY", "DataType"=bool[] [] ("appended array")) -> ("data out"=w247:bool[])  [unwired: 6 in, 6 out]
        n100 = Index Array(array=w247, index #1=5 ("index")) -> (element #1=w245:bool, element #2=w244:bool, element #3=w243:bool, element #4=w242:bool, element #5=w241:bool, element #6=w240:bool, element #7=w239:bool, element #8=w238:bool, element #9=w237:bool, element #10=w236:bool, element #11=w235:bool, element #12=w234:bool, element #13=w233:bool, element #14=→"DO 18":bool)  [unwired: 13 in]
        n101 = Not(x=w245) -> (.not. x?=→"DO 5":bool)
        n102 = Not(x=w244) -> (.not. x?=→"DO 6":bool)
        n103 = Not(x=w243) -> (.not. x?=→"DO 7":bool)
        n104 = Not(x=w242) -> (.not. x?=→"DO 8":bool)
        n105 = Not(x=w241) -> (.not. x?=→"DO 9":bool)
        n106 = Not(x=w240) -> (.not. x?=→"DO 10":bool)
        n107 = Not(x=w239) -> (.not. x?=→"DO 11":bool)
        n108 = Not(x=w238) -> (.not. x?=→"DO 12":bool)
        n109 = Not(x=w237) -> (.not. x?=→"DO 13":bool)
        n110 = Not(x=w236) -> (.not. x?=→"DO 14":bool)
        n111 = Not(x=w235) -> (.not. x?=→"DO 15":bool)
        n112 = Not(x=w234) -> (.not. x?=→"DO 16":bool)
        n113 = Not(x=w233) -> (.not. x?=→"DO 17":bool)
      }
      frame #10 {
        n114 = call "Read.vim"("SharedVariableWrapper in"=w251, "name"="STATE_PMG", "DataType"=T30 {"PMG Mode"=enum."Idel", "M12"={"EngState"=enum."Unknown", "Active"=FALSE, "Contactor"=FALSE, "CMD"=FALSE, "Automat"=FALSE}, "M21"={"EngState"=enum."Unknown", "Active"=FALSE, "Contactor"=FALSE, "CMD"=FALSE, "Automat"=FALSE}, "M24"={"EngState"=enum."Unknown", "Active"=FALSE, "Contactor"=FALSE, "CMD"=FALSE, "Automat"=FALSE}} ("PMG")) -> ("data out"=w255:T30)  [unwired: 6 in, 6 out]
        n115 = Unbundle By Name(w255) -> ("M12"=→"m12":T32, "M21"=→"m21":T32, "M24"=→"m24":T32)
      }
      frame #11 {
        n116 = call "Read.vim"("SharedVariableWrapper in"=w263, "name"="AO_ARRAY", "DataType"=dbl[] [] ("appended array")) -> ("data out"=w260:dbl[])  [unwired: 6 in, 6 out]
        n117 = Index Array(array=w260) -> (element #1=→"AO 0":dbl, element #2=→"AO 1":dbl)  [unwired: 2 in]
      }
    }
    n118 = Bundle("SP DUT"=w18, "scl mean 1Hz"=w16, "scl mean 1Hz"=w14) -> (→"dut":T33)  [unwired: 1 in]
    n119 = Bundle("SP CHAMBER"=w17, "scl mean 1Hz"=w15, "scl mean 1Hz"=w13) -> (→"chmbr":T34)  [unwired: 1 in]
    n120 = Merge Errors(w27, w28, w32, w31, w26, w25, w21, w12) -> (w30:errorcluster)
    n121 = Wait Until Next ms Multiple(millisecond multiple=u32 200) -> (millisecond timer value=w24:u32)
    n122 = Unbundle By Name(w30) -> ("status"=→"Connect":bool)
  }
  n123 = while {
    shift-right: [w270] -> _
    shift-left: _ -> [w269]
    shift-right: [w273] -> w7
    shift-left: w3 -> [w267]
    shift-right: [w272] -> _
    shift-left: w9 -> [w274]
    tunnel: w1 -> [w266]
    shift-right: [w265] -> _
    shift-left: _ -> [w264]
    stop <- w271 stop-if-true
    w268 = -1  # Timeout
    n124 = call <vilib>:"Parse State Queue__JKI_lib_State_Machine.vi"("State Queue"=w274, "Error In (no error)"=w267) -> ("Remaining States"=w276:string, "Current State"=w277:string, "Arguments"=w275:string)  [unwired: 11 in]
    n125 = case shown="\"\", \"Event Structure\", \"Idle\"" w277 {
      selector: w277 -> [_ _ w707 _ _ _ _ _ _ _ _ _ _ _ _ _ _ _ _ _ _ _ _ _ _]
      tunnel: w276 -> [w286 w705 w711 w731 w738 w744 w749 w758 w765 w770 w777 w783 w788 w793 w800 w812 w882 w888 w894 w906 w910 w911 w918 w922 w924]
      tunnel: w275 -> [_ _ _ _ _ _ _ _ _ _ _ _ _ _ w795 w806 _ _ _ _ _ _ _ _ _]
      tunnel: w269 -> [w284 w702 w709 w724 w735 w742 w746 _ w760 w767 w776 w781 w785 w792 w798 w808 w879 w885 w891 w903 w908 w912 w915 w919 w923]
      tunnel: [w283 w703 w713 w728 errorcluster {"status"=FALSE, "code"=0, "source"=""} ("error out") w741 w747 w750 w761 w768 w774 w778 w786 w791 w796 w809 w880 w886 w892 w904 w909 w913 w916 w920 w926] -> w273
      tunnel: w267 -> [w282 w703 w712 w728 w734 w741 w747 w752 w762 w768 w773 w779 w786 w791 w797 w810 w880 w886 w892 w904 w909 w913 w916 w920 w926]
      tunnel: [w285 w704 w710 w730 w737 w743 w748 w758 w764 w769 w777 w782 w787 w793 w799 w811 w881 w887 w893 w905 w910 w911 w918 w922 w924] -> w272
      tunnel: [_ _ _ _ _ TRUE _ _ _ _ _ _ _ _ _ _ _ _ _ _ _ _ _ _ _] -> w271
      tunnel: [w281 w702 w709 w729 w735 w742 w746 w757 w760 w767 w776 w781 w785 w792 w798 w808 w879 w885 w891 w903 w908 w912 w915 w919 w923] -> w270
      tunnel: w268 -> [w280 _ _ _ _ _ _ _ _ _ _ _ _ _ _ _ _ _ _ _ _ _ _ _ _]
      tunnel: w266 -> [w279 _ _ _ _ _ _ _ _ _ w772 _ _ _ _ _ _ _ _ _ _ _ _ _ _]
      tunnel: [w278 w701 w706 w718 w732 w739 w745 w755 w759 w766 w775 w780 w784 w790 w794 w805 w878 w883 w889 w896 w907 w914 w917 w921 w925] -> w265
      tunnel: w264 -> [w278 w701 w706 w718 w732 w739 w745 w755 w759 w766 _ w780 w784 w790 w794 w805 w878 w883 w889 w896 w907 w914 w917 w921 w925]
      frame "", "Event Structure", "Idle" {
        n126 = event shown="[13] \"alarm press\": Value Change" {
          selector: w278 -> [_ _ _ _ _ _ _ _ _ _ _ _ _ _ _]
          dyn-events: _ -> [_ _ _ _ _ _ _ _ _ _ _ _ _ _ _]
          timeout: w280 -> [_ _ _ _ _ _ _ _ _ _ _ _ _ _ _]
          tunnel: w286 -> [w290 w298 w305 w319 w328 w336 w354 w371 w411 w458 w517 w568 w623 w686 w700]
          tunnel: [w289 w297 w304 w319 w328 w336 w354 w371 w411 w458 w517 w568 w623 w686 w700] -> w285
          tunnel: w284 -> [w287 w296 w303 w308 w327 w335 w353 w367 w407 w449 w508 w567 w622 w675 w690]
          tunnel: [w288 w291 w299 w306 w320 w330 w348 w370 w410 w446 w505 w564 w619 w673 w687] -> w283
          tunnel: w282 -> [w288 w292 w300 w307 w321 w331 w349 w370 w410 w447 w506 w565 w620 w674 w688]
          tunnel: [w287 w296 w303 w308 w327 w335 w353 w367 w407 w449 w508 w567 w622 w675 w690] -> w281
          tunnel: w279 -> [_ w293 w301 w309 _ _ _ w368 w408 w448 w507 w566 w621 w676 w689]
          event Timeout {
            n127 = event-data() -> ()  [unwired: 1 in, 1 out]
            n128 = call <vilib>:"Add State(s) to Queue__JKI_lib_State_Machine.vi"("State(s) in (\"\")"=w290) -> ("States Out"=w289:string)  [unwired: 14 in]
          }
          event Panel Close? {
            n129 = event-data() -> ()  [unwired: 1 in, 1 out]
            n130 = call "CMD_Close.vi"("reference in"=w293, "error in (no error)"=w292) -> ("error out"=w291:errorcluster)  [unwired: 12 in, 1 out]
            n131 = call <vilib>:"Add State(s) to Queue__JKI_lib_State_Machine.vi"("State(s) in Front (\"\")"="// Macro: Exit", "State(s) in (\"\")"=w298) -> ("States Out"=w297:string)  [unwired: 13 in]
            n132 = event-data("Discard?"=TRUE) -> ()  [unwired: 1 in, 1 out]
          }
          event User Event {
            n133 = event-data() -> ()  [unwired: 1 in, 5 out]
            n134 = call "CMD_Close.vi"("reference in"=w301, "error in (no error)"=w300) -> ("error out"=w299:errorcluster)  [unwired: 12 in, 1 out]
            n135 = call <vilib>:"Add State(s) to Queue__JKI_lib_State_Machine.vi"("State(s) in Front (\"\")"="Macro: Exit", "State(s) in (\"\")"=w305) -> ("States Out"=w304:string)  [unwired: 13 in]
          }
          event "Clear Error": Value Change {
            n136 = event-data() -> ()  [unwired: 1 in, 6 out]
            n137 = Unbundle By Name(w308) -> ("amc"=w318:refnum<class "MessageAMC.lvclass">)
            n138 = call "Read SVW.vi"("GUI in"=w309) -> ("SharedVariableWrapper.lvclass"=w313:refnum<class "SharedVariableWrapper.lvclass">)  [unwired: 10 in]
            n139 = call "ReadConfig.vi"("SharedVariableWrapper in"=w313) -> ("config"=w312:T38)  [unwired: 12 in, 2 out]
            n140 = Unbundle By Name(w312) -> ("ip"=w311:string)
            n141 = call "SendNetworkVariant.vi"("reference in"=w318, "receiver process"="STAND", "receiver host"=w311, "receiver port (0)"=u16 54321, "name"="RESET_ALARMS", "data"=TRUE, "timeout (25000 ms)"=1000, "error in (no error)"=w307) -> ("error out"=w306:errorcluster)  [unwired: 5 in, 2 out]
          }
          event "DO 5", "DO 9", "DO 10", "DO 17", "DO 12", "DO 13", "DO 15", "DO 16", "DO 14", "44.2", "44.1", "DO 18", "DO 8", "DO 11", "DO 6", "DO 7": Shortcut Menu Activation? {
            n142 = event-data() -> ("MenuRef"=w326:refnum<k9>)  [unwired: 1 in, 6 out]
            n143 = Delete Menu Items(6:w321, 9:w326) -> (0:w324:errorcluster, 3:w325:refnum<k9>)  [unwired: 2 in]
            n144 = Insert Menu Items(6:w324, 7:string[] ["open", "close"] ("item tags"), 8:string[] ["Открыть", "Закрыть"] ("item names"), 9:w325) -> (0:w320:errorcluster)  [unwired: 2 in, 2 out]
            n145 = event-data() -> ()  [unwired: 2 in, 1 out]
          }
          event "37.1": Shortcut Menu Activation? {
            n146 = event-data() -> ("MenuRef"=w334:refnum<k9>)  [unwired: 1 in, 6 out]
            n147 = Delete Menu Items(6:w331, 9:w334) -> (0:w332:errorcluster, 3:w333:refnum<k9>)  [unwired: 2 in]
            n148 = local read "StateValveModbus"() -> (w329:T2)
            n149 = case shown="Default" w329 {
              tunnel: w333 -> [w341 w346]
              tunnel: w332 -> [w340 w345]
              tunnel: [w337 w342] -> w330
              frame Default {
                n150 = Insert Menu Items(6:w340, 7:string[] ["open", "close"] ("item tags"), 8:string[] ["Открыть", "Закрыть"] ("item names"), 9:w341) -> (0:w337:errorcluster)  [unwired: 2 in, 2 out]
              }
              frame "OPENING", "CLOSING" {
                n151 = Insert Menu Items(6:w345, 7:string[] ["stop"] ("item tags"), 8:string[] ["Стоп"] ("item names"), 9:w346) -> (0:w342:errorcluster)  [unwired: 2 in, 2 out]
              }
            }
            n152 = event-data() -> ()  [unwired: 2 in, 1 out]
          }
          event "37.2": Shortcut Menu Activation? {
            n153 = event-data() -> ("MenuRef"=w352:refnum<k9>)  [unwired: 1 in, 6 out]
            n154 = local read "StateValveModbus 2"() -> (w347:T2)
            n155 = Delete Menu Items(6:w349, 9:w352) -> (0:w350:errorcluster, 3:w351:refnum<k9>)  [unwired: 2 in]
            n156 = case shown="Default" w347 {
              tunnel: w351 -> [w359 w364]
              tunnel: w350 -> [w358 w363]
              tunnel: [w355 w360] -> w348
              frame Default {
                n157 = Insert Menu Items(6:w358, 7:string[] ["open", "close"] ("item tags"), 8:string[] ["Открыть", "Закрыть"] ("item names"), 9:w359) -> (0:w355:errorcluster)  [unwired: 2 in, 2 out]
              }
              frame "OPENING", "CLOSING" {
                n158 = Insert Menu Items(6:w363, 7:string[] ["stop"] ("item tags"), 8:string[] ["Стоп"] ("item names"), 9:w364) -> (0:w360:errorcluster)  [unwired: 2 in, 2 out]
              }
            }
            n159 = event-data() -> ()  [unwired: 2 in, 1 out]
          }
          event "37.1": Shortcut Menu Selection (User) {
            n160 = event-data() -> ("ItemTag"=w366:string)  [unwired: 1 in]
            n161 = Unbundle By Name(w367) -> ("amc"=w369:refnum<class "MessageAMC.lvclass">)
            n162 = case shown="\"stop\"" w366 {
              tunnel: w369 -> [_ w377 w388 w399]
              tunnel: w368 -> [_ w373 w384 w395]
              tunnel: "NV1" ("receiver process") -> [_ w372 w383 w394]
              frame "False", Default {
              }
              frame "open" {
                n163 = call "Read SVW.vi"("GUI in"=w373) -> ("SharedVariableWrapper.lvclass"=w379:refnum<class "SharedVariableWrapper.lvclass">)  [unwired: 10 in]
                n164 = call "ReadConfig.vi"("SharedVariableWrapper in"=w379) -> ("config"=w378:T38)  [unwired: 12 in, 2 out]
                n165 = Unbundle By Name(w378) -> ("ip"=w376:string)
                n166 = call "SendNetworkVariant.vi"("reference in"=w377, "receiver process"=w372, "receiver host"=w376, "receiver port (0)"=u16 54321, "name"="OPEN", "data"=FALSE, "timeout (25000 ms)"=1000) -> ("error out"=w374:errorcluster)  [unwired: 6 in, 2 out]
                n167 = call <vilib>:"Simple Error Handler.vi"("error in (no error)"=w374) -> ()  [unwired: 4 in, 5 out]
              }
              frame "close" {
                n168 = call "Read SVW.vi"("GUI in"=w384) -> ("SharedVariableWrapper.lvclass"=w390:refnum<class "SharedVariableWrapper.lvclass">)  [unwired: 10 in]
                n169 = call "ReadConfig.vi"("SharedVariableWrapper in"=w390) -> ("config"=w389:T38)  [unwired: 12 in, 2 out]
                n170 = Unbundle By Name(w389) -> ("ip"=w387:string)
                n171 = call "SendNetworkVariant.vi"("reference in"=w388, "receiver process"=w383, "receiver host"=w387, "receiver port (0)"=u16 54321, "name"="CLOSE", "data"=FALSE, "timeout (25000 ms)"=1000) -> ("error out"=w385:errorcluster)  [unwired: 6 in, 2 out]
                n172 = call <vilib>:"Simple Error Handler.vi"("error in (no error)"=w385) -> ()  [unwired: 4 in, 5 out]
              }
              frame "stop" {
                n173 = call "Read SVW.vi"("GUI in"=w395) -> ("SharedVariableWrapper.lvclass"=w401:refnum<class "SharedVariableWrapper.lvclass">)  [unwired: 10 in]
                n174 = call "ReadConfig.vi"("SharedVariableWrapper in"=w401) -> ("config"=w400:T38)  [unwired: 12 in, 2 out]
                n175 = Unbundle By Name(w400) -> ("ip"=w398:string)
                n176 = call "SendNetworkVariant.vi"("reference in"=w399, "receiver process"=w394, "receiver host"=w398, "receiver port (0)"=u16 54321, "name"="STOP", "data"=FALSE, "timeout (25000 ms)"=1000) -> ("error out"=w396:errorcluster)  [unwired: 6 in, 2 out]
                n177 = call <vilib>:"Simple Error Handler.vi"("error in (no error)"=w396) -> ()  [unwired: 4 in, 5 out]
              }
            }
          }
          event "37.2": Shortcut Menu Selection (User) {
            n178 = event-data() -> ("ItemTag"=w406:string)  [unwired: 1 in]
            n179 = Unbundle By Name(w407) -> ("amc"=w409:refnum<class "MessageAMC.lvclass">)
            n180 = case shown="\"stop\"" w406 {
              tunnel: w409 -> [_ w417 w428 w439]
              tunnel: w408 -> [_ w413 w424 w435]
              tunnel: "NV2" ("receiver process") -> [_ w412 w423 w434]
              frame "False", Default {
              }
              frame "open" {
                n181 = call "Read SVW.vi"("GUI in"=w413) -> ("SharedVariableWrapper.lvclass"=w419:refnum<class "SharedVariableWrapper.lvclass">)  [unwired: 10 in]
                n182 = call "ReadConfig.vi"("SharedVariableWrapper in"=w419) -> ("config"=w418:T38)  [unwired: 12 in, 2 out]
                n183 = Unbundle By Name(w418) -> ("ip"=w416:string)
                n184 = call "SendNetworkVariant.vi"("reference in"=w417, "receiver process"=w412, "receiver host"=w416, "receiver port (0)"=u16 54321, "name"="OPEN", "data"=FALSE, "timeout (25000 ms)"=1000) -> ("error out"=w414:errorcluster)  [unwired: 6 in, 2 out]
                n185 = call <vilib>:"Simple Error Handler.vi"("error in (no error)"=w414) -> ()  [unwired: 4 in, 5 out]
              }
              frame "close" {
                n186 = call "Read SVW.vi"("GUI in"=w424) -> ("SharedVariableWrapper.lvclass"=w430:refnum<class "SharedVariableWrapper.lvclass">)  [unwired: 10 in]
                n187 = call "ReadConfig.vi"("SharedVariableWrapper in"=w430) -> ("config"=w429:T38)  [unwired: 12 in, 2 out]
                n188 = Unbundle By Name(w429) -> ("ip"=w427:string)
                n189 = call "SendNetworkVariant.vi"("reference in"=w428, "receiver process"=w423, "receiver host"=w427, "receiver port (0)"=u16 54321, "name"="CLOSE", "data"=FALSE, "timeout (25000 ms)"=1000) -> ("error out"=w425:errorcluster)  [unwired: 6 in, 2 out]
                n190 = call <vilib>:"Simple Error Handler.vi"("error in (no error)"=w425) -> ()  [unwired: 4 in, 5 out]
              }
              frame "stop" {
                n191 = call "Read SVW.vi"("GUI in"=w435) -> ("SharedVariableWrapper.lvclass"=w441:refnum<class "SharedVariableWrapper.lvclass">)  [unwired: 10 in]
                n192 = call "ReadConfig.vi"("SharedVariableWrapper in"=w441) -> ("config"=w440:T38)  [unwired: 12 in, 2 out]
                n193 = Unbundle By Name(w440) -> ("ip"=w438:string)
                n194 = call "SendNetworkVariant.vi"("reference in"=w439, "receiver process"=w434, "receiver host"=w438, "receiver port (0)"=u16 54321, "name"="STOP", "data"=FALSE, "timeout (25000 ms)"=1000) -> ("error out"=w436:errorcluster)  [unwired: 6 in, 2 out]
                n195 = call <vilib>:"Simple Error Handler.vi"("error in (no error)"=w436) -> ()  [unwired: 4 in, 5 out]
              }
            }
          }
          event "DO 5", "DO 9", "DO 10", "DO 17", "DO 12", "DO 13", "DO 15", "DO 16", "DO 14", "DO 8", "DO 11", "DO 6", "DO 7": Shortcut Menu Selection (User) {
            n196 = event-data() -> ("CtlRef"=w450:refnum<vi>, "ItemTag"=w445:string)  [unwired: 1 in, 6 out]
            n197 = property class="Bool (strict)"(reference=w450) -> ("Label.Text"=w453:string)  [unwired: 1 in, 2 out]
            n198 = Match Pattern(string=w453, regular expression="[0-9]+") -> (match substring=w454:string, offset past match=w456:i32)  [unwired: 1 in, 2 out]
            n199 = Not Equal?(x=w456, y=-1) -> (x != y?=w452:bool)
            n200 = Decimal String To Number(string=w454) -> (number=w451:i32)  [unwired: 2 in, 1 out]
            n201 = case shown="Default" w445 {
              tunnel: w452 -> [_ w465 w487]
              tunnel: w451 -> [_ w464 w486]
              tunnel: w449 -> [_ w463 w485]
              tunnel: w448 -> [_ w462 w484]
              tunnel: w447 -> [w459 w461 w483]
              tunnel: [w459 w460 w482] -> w446
              frame Default {
              }
              frame "open" {
                n202 = case shown="True" w465 {
                  tunnel: w463 -> [_ w481]
                  tunnel: w462 -> [_ w480]
                  tunnel: w461 -> [w466 w479]
                  tunnel: [w466 w478] -> w460
                  tunnel: w464 -> [_ w469]
                  frame False {
                  }
                  frame True {
                    n203 = Unbundle By Name(w481) -> ("amc"=w477:refnum<class "MessageAMC.lvclass">)
                    n204 = call "Read SVW.vi"("GUI in"=w480) -> ("SharedVariableWrapper.lvclass"=w472:refnum<class "SharedVariableWrapper.lvclass">)  [unwired: 10 in]
                    n205 = Bundle(w469, FALSE) -> (w468:cluster{i32, bool})  [unwired: 1 in]
                    n206 = call "ReadConfig.vi"("SharedVariableWrapper in"=w472) -> ("config"=w471:T38)  [unwired: 12 in, 2 out]
                    n207 = Unbundle By Name(w471) -> ("ip"=w470:string)
                    n208 = call "SendNetworkVariant.vi"("reference in"=w477, "receiver process"="STAND", "receiver host"=w470, "receiver port (0)"=u16 54321, "name"="SET_DO", "data"=w468, "timeout (25000 ms)"=1000, "error in (no error)"=w479) -> ("error out"=w478:errorcluster)  [unwired: 5 in, 2 out]
                  }
                }
              }
              frame "close" {
                n209 = case shown="True" w487 {
                  tunnel: w485 -> [_ w503]
                  tunnel: w484 -> [_ w502]
                  tunnel: w483 -> [w488 w501]
                  tunnel: [w488 w500] -> w482
                  tunnel: w486 -> [_ w491]
                  frame False {
                  }
                  frame True {
                    n210 = Unbundle By Name(w503) -> ("amc"=w499:refnum<class "MessageAMC.lvclass">)
                    n211 = call "Read SVW.vi"("GUI in"=w502) -> ("SharedVariableWrapper.lvclass"=w494:refnum<class "SharedVariableWrapper.lvclass">)  [unwired: 10 in]
                    n212 = Bundle(w491, TRUE) -> (w490:cluster{i32, bool})  [unwired: 1 in]
                    n213 = call "ReadConfig.vi"("SharedVariableWrapper in"=w494) -> ("config"=w493:T38)  [unwired: 12 in, 2 out]
                    n214 = Unbundle By Name(w493) -> ("ip"=w492:string)
                    n215 = call "SendNetworkVariant.vi"("reference in"=w499, "receiver process"="STAND", "receiver host"=w492, "receiver port (0)"=u16 54321, "name"="SET_DO", "data"=w490, "timeout (25000 ms)"=1000, "error in (no error)"=w501) -> ("error out"=w500:errorcluster)  [unwired: 5 in, 2 out]
                  }
                }
              }
            }
          }
          event "DO 18": Shortcut Menu Selection (User) {
            n216 = event-data() -> ("CtlRef"=w509:refnum<vi>, "ItemTag"=w504:string)  [unwired: 1 in, 6 out]
            n217 = property class="Bool (strict)"(reference=w509) -> ("Label.Text"=w512:string)  [unwired: 1 in, 2 out]
            n218 = Match Pattern(string=w512, regular expression="[0-9]+") -> (match substring=w513:string, offset past match=w515:i32)  [unwired: 1 in, 2 out]
            n219 = Not Equal?(x=w515, y=-1) -> (x != y?=w511:bool)
            n220 = Decimal String To Number(string=w513) -> (number=w510:i32)  [unwired: 2 in, 1 out]
            n221 = case shown="\"close\"" w504 {
              tunnel: w511 -> [_ w524 w546]
              tunnel: w510 -> [_ w523 w545]
              tunnel: w508 -> [_ w522 w544]
              tunnel: w507 -> [_ w521 w543]
              tunnel: w506 -> [w518 w520 w542]
              tunnel: [w518 w519 w541] -> w505
              frame Default {
              }
              frame "open" {
                n222 = case shown="True" w524 {
                  tunnel: w522 -> [_ w540]
                  tunnel: w521 -> [_ w539]
                  tunnel: w520 -> [w525 w538]
                  tunnel: [w525 w537] -> w519
                  tunnel: w523 -> [_ w528]
                  frame False {
                  }
                  frame True {
                    n223 = Unbundle By Name(w540) -> ("amc"=w536:refnum<class "MessageAMC.lvclass">)
                    n224 = call "Read SVW.vi"("GUI in"=w539) -> ("SharedVariableWrapper.lvclass"=w531:refnum<class "SharedVariableWrapper.lvclass">)  [unwired: 10 in]
                    n225 = Bundle(w528, TRUE) -> (w527:cluster{i32, bool})  [unwired: 1 in]
                    n226 = call "ReadConfig.vi"("SharedVariableWrapper in"=w531) -> ("config"=w530:T38)  [unwired: 12 in, 2 out]
                    n227 = Unbundle By Name(w530) -> ("ip"=w529:string)
                    n228 = call "SendNetworkVariant.vi"("reference in"=w536, "receiver process"="STAND", "receiver host"=w529, "receiver port (0)"=u16 54321, "name"="SET_DO", "data"=w527, "timeout (25000 ms)"=1000, "error in (no error)"=w538) -> ("error out"=w537:errorcluster)  [unwired: 5 in, 2 out]
                  }
                }
              }
              frame "close" {
                n229 = case shown="True" w546 {
                  tunnel: w544 -> [_ w562]
                  tunnel: w543 -> [_ w561]
                  tunnel: w542 -> [w547 w560]
                  tunnel: [w547 w559] -> w541
                  tunnel: w545 -> [_ w550]
                  frame False {
                  }
                  frame True {
                    n230 = Unbundle By Name(w562) -> ("amc"=w558:refnum<class "MessageAMC.lvclass">)
                    n231 = call "Read SVW.vi"("GUI in"=w561) -> ("SharedVariableWrapper.lvclass"=w553:refnum<class "SharedVariableWrapper.lvclass">)  [unwired: 10 in]
                    n232 = Bundle(w550, FALSE) -> (w549:cluster{i32, bool})  [unwired: 1 in]
                    n233 = call "ReadConfig.vi"("SharedVariableWrapper in"=w553) -> ("config"=w552:T38)  [unwired: 12 in, 2 out]
                    n234 = Unbundle By Name(w552) -> ("ip"=w551:string)
                    n235 = call "SendNetworkVariant.vi"("reference in"=w558, "receiver process"="STAND", "receiver host"=w551, "receiver port (0)"=u16 54321, "name"="SET_DO", "data"=w549, "timeout (25000 ms)"=1000, "error in (no error)"=w560) -> ("error out"=w559:errorcluster)  [unwired: 5 in, 2 out]
                  }
                }
              }
            }
          }
          event "44.1": Shortcut Menu Selection (User) {
            n236 = event-data() -> ("ItemTag"=w563:string)  [unwired: 1 in, 7 out]
            n237 = case shown="\"open\"" w563 {
              tunnel: w567 -> [_ w580 w604]
              tunnel: w566 -> [_ w579 w603]
              tunnel: w565 -> [w569 w578 w602]
              tunnel: [w569 w577 w601] -> w564
              frame Default {
              }
              frame "close" {
                n238 = Bundle(21, TRUE) -> (w571:cluster{i32, bool})  [unwired: 1 in]
                n239 = Bundle(20, FALSE) -> (w572:cluster{i32, bool})  [unwired: 1 in]
                n240 = Build Array(w572, w571) -> (w570:cluster{i32, bool}[])
                n241 = for {
                  tunnel: w580 -> [w593]
                  tunnel: w579 -> [w592]
                  shift-right: [w590] -> w577
                  shift-left: w578 -> [w591]
                  tunnel: w570 -> [w581] mode=indexing
                  n242 = Unbundle By Name(w593) -> ("amc"=w589:refnum<class "MessageAMC.lvclass">)
                  n243 = call "Read SVW.vi"("GUI in"=w592) -> ("SharedVariableWrapper.lvclass"=w584:refnum<class "SharedVariableWrapper.lvclass">)  [unwired: 10 in]
                  n244 = call "ReadConfig.vi"("SharedVariableWrapper in"=w584) -> ("config"=w583:T38)  [unwired: 12 in, 2 out]
                  n245 = Unbundle By Name(w583) -> ("ip"=w582:string)
                  n246 = call "SendNetworkVariant.vi"("reference in"=w589, "receiver process"="STAND", "receiver host"=w582, "receiver port (0)"=u16 54321, "name"="SET_DO", "data"=w581, "timeout (25000 ms)"=1000, "error in (no error)"=w591) -> ("error out"=w590:errorcluster)  [unwired: 5 in, 2 out]
                }
              }
              frame "open" {
                n247 = Bundle(20, TRUE) -> (w595:cluster{i32, bool})  [unwired: 1 in]
                n248 = Bundle(21, FALSE) -> (w596:cluster{i32, bool})  [unwired: 1 in]
                n249 = Build Array(w596, w595) -> (w594:cluster{i32, bool}[])
                n250 = for {
                  tunnel: w604 -> [w617]
                  tunnel: w603 -> [w616]
                  shift-right: [w614] -> w601
                  shift-left: w602 -> [w615]
                  tunnel: w594 -> [w605] mode=indexing
                  n251 = Unbundle By Name(w617) -> ("amc"=w613:refnum<class "MessageAMC.lvclass">)
                  n252 = call "Read SVW.vi"("GUI in"=w616) -> ("SharedVariableWrapper.lvclass"=w608:refnum<class "SharedVariableWrapper.lvclass">)  [unwired: 10 in]
                  n253 = call "ReadConfig.vi"("SharedVariableWrapper in"=w608) -> ("config"=w607:T38)  [unwired: 12 in, 2 out]
                  n254 = Unbundle By Name(w607) -> ("ip"=w606:string)
                  n255 = call "SendNetworkVariant.vi"("reference in"=w613, "receiver process"="STAND", "receiver host"=w606, "receiver port (0)"=u16 54321, "name"="SET_DO", "data"=w605, "timeout (25000 ms)"=1000, "error in (no error)"=w615) -> ("error out"=w614:errorcluster)  [unwired: 5 in, 2 out]
                }
              }
            }
          }
          event "44.2": Shortcut Menu Selection (User) {
            n256 = event-data() -> ("ItemTag"=w618:string)  [unwired: 1 in, 7 out]
            n257 = case shown="\"close\"" w618 {
              tunnel: w622 -> [_ w635 w659]
              tunnel: w621 -> [_ w634 w658]
              tunnel: w620 -> [w624 w633 w657]
              tunnel: [w624 w632 w656] -> w619
              frame Default {
              }
              frame "close" {
                n258 = Bundle(23, TRUE) -> (w626:cluster{i32, bool})  [unwired: 1 in]
                n259 = Bundle(22, FALSE) -> (w627:cluster{i32, bool})  [unwired: 1 in]
                n260 = Build Array(w627, w626) -> (w625:cluster{i32, bool}[])
                n261 = for {
                  tunnel: w635 -> [w648]
                  tunnel: w634 -> [w647]
                  shift-right: [w645] -> w632
                  shift-left: w633 -> [w646]
                  tunnel: w625 -> [w636] mode=indexing
                  n262 = Unbundle By Name(w648) -> ("amc"=w644:refnum<class "MessageAMC.lvclass">)
                  n263 = call "Read SVW.vi"("GUI in"=w647) -> ("SharedVariableWrapper.lvclass"=w639:refnum<class "SharedVariableWrapper.lvclass">)  [unwired: 10 in]
                  n264 = call "ReadConfig.vi"("SharedVariableWrapper in"=w639) -> ("config"=w638:T38)  [unwired: 12 in, 2 out]
                  n265 = Unbundle By Name(w638) -> ("ip"=w637:string)
                  n266 = call "SendNetworkVariant.vi"("reference in"=w644, "receiver process"="STAND", "receiver host"=w637, "receiver port (0)"=u16 54321, "name"="SET_DO", "data"=w636, "timeout (25000 ms)"=1000, "error in (no error)"=w646) -> ("error out"=w645:errorcluster)  [unwired: 5 in, 2 out]
                }
              }
              frame "open" {
                n267 = Bundle(22, TRUE) -> (w650:cluster{i32, bool})  [unwired: 1 in]
                n268 = Bundle(23, FALSE) -> (w651:cluster{i32, bool})  [unwired: 1 in]
                n269 = Build Array(w651, w650) -> (w649:cluster{i32, bool}[])
                n270 = for {
                  tunnel: w659 -> [w672]
                  tunnel: w658 -> [w671]
                  shift-right: [w669] -> w656
                  shift-left: w657 -> [w670]
                  tunnel: w649 -> [w660] mode=indexing
                  n271 = Unbundle By Name(w672) -> ("amc"=w668:refnum<class "MessageAMC.lvclass">)
                  n272 = call "Read SVW.vi"("GUI in"=w671) -> ("SharedVariableWrapper.lvclass"=w663:refnum<class "SharedVariableWrapper.lvclass">)  [unwired: 10 in]
                  n273 = call "ReadConfig.vi"("SharedVariableWrapper in"=w663) -> ("config"=w662:T38)  [unwired: 12 in, 2 out]
                  n274 = Unbundle By Name(w662) -> ("ip"=w661:string)
                  n275 = call "SendNetworkVariant.vi"("reference in"=w668, "receiver process"="STAND", "receiver host"=w661, "receiver port (0)"=u16 54321, "name"="SET_DO", "data"=w660, "timeout (25000 ms)"=1000, "error in (no error)"=w670) -> ("error out"=w669:errorcluster)  [unwired: 5 in, 2 out]
                }
              }
            }
          }
          event "alarm press": Value Change {
            n276 = event-data() -> ()  [unwired: 1 in, 6 out]
            n277 = call "Read SVW.vi"("GUI in"=w676) -> ("SharedVariableWrapper.lvclass"=w685:refnum<class "SharedVariableWrapper.lvclass">)  [unwired: 10 in]
            n278 = Unbundle By Name(w675) -> ("amc"=w677:refnum<class "MessageAMC.lvclass">)
            n279 = call "ReadConfig.vi"("SharedVariableWrapper in"=w685) -> ("config"=w684:T38)  [unwired: 12 in, 2 out]
            n280 = Unbundle By Name(w684) -> ("ip"=w683:string)
            n281 = call "SendNetworkVariant.vi"("reference in"=w677, "receiver process"="STAND", "receiver host"=w683, "receiver port (0)"=u16 54321, "name"="CMD", "data"=T35 {"EXECUTE_SP"=FALSE, "ALARM_PRESS_DOWN_DUT"=FALSE, "ALARM_PRESS_DOWN_CHAMBER"=FALSE, "ALARM_PRESS_DOWN_DUT_CHAMBER"=TRUE, "FILING_DUT"=FALSE, "FILING_CHAMBER"=FALSE, "BLOCK"=FALSE, "PUMP_STATION_OFF"=FALSE, "OPEN_44_2"=FALSE, "CLOSE_44_2"=FALSE, "Drain"=FALSE} ("CMD REG"), "timeout (25000 ms)"=1000, "error in (no error)"=w674) -> ("error out"=w673:errorcluster)  [unwired: 5 in, 2 out]
          }
          event "remote": Value Change {
            n282 = event-data() -> ()  [unwired: 1 in, 6 out]
            n283 = call "Read SVW.vi"("GUI in"=w689) -> ("SharedVariableWrapper.lvclass"=w695:refnum<class "SharedVariableWrapper.lvclass">)  [unwired: 10 in]
            n284 = call "ReadConfig.vi"("SharedVariableWrapper in"=w695) -> ("config"=w696:T38)  [unwired: 12 in, 2 out]
            n285 = Unbundle By Name(w696) -> ("ip"=w697:string)
            n286 = Unbundle By Name(w690) -> ("amc"=w698:refnum<class "MessageAMC.lvclass">)
            n287 = call "SendNetworkVariant.vi"("reference in"=w698, "receiver process"="STAND", "receiver host"=w697, "receiver port (0)"=u16 54321, "name"="SET_REMOTE", "data"="remote", "timeout (25000 ms)"=1000, "error in (no error)"=w688) -> ("error out"=w687:errorcluster)  [unwired: 5 in, 2 out]
          }
        }
      }
      frame "---------- Core ----------" {
        n288 = call <vilib>:"Add State(s) to Queue__JKI_lib_State_Machine.vi"("State(s) in (\"\")"=w705) -> ("States Out"=w704:string)  [unwired: 14 in]
      }
      frame Default {
        w716 = 42 items=["No error", "Argument error", "Memory is full", "Out of zone", "End of file", "File already open", "Generic file I/O error", "File not found", "File permission error", "Disk is full", "Duplicate path", "Too many files open", "System feature not enabled", "Resource file not found", "Cannot add resource", "Resource not found", "Image not found", "Image memory error", "Pen does not exist", "Config type invalid", "Config token not found", "Config parse error", "Config memory error", "Bad external code format", "Bad external code offset", "External code not present", "Null window", "Destroy window error", "Null menu", "Print aborted", "Bad print record", "Print driver error", "Windows error during printing", "Memory error during printing", "Print dialog error", "Generic print error", "Invalid device refnum", "Device not found", "Device parameter error", "Device unit error", "Cannot open device", "Device call aborted", "Generic error", "Cancelled by user", "Object ID too low", "Object ID too high", "Object not in heap", "Unknown heap", "Unknown object (invalid DefProc)", "Unknown object (DefProc not in table)", "Message out of range", "Invalid (null) method", "Unknown message", "Manager call not supported", "Bad address", "Network operation in progress", "Network operation timed out", "Connection is busy", "Network attribute not supported", "Network error", "Address in use", "System out of memory", "Connection aborted", "Connection refused", "Not connected", "Already connected", "Connection closed", "Initialization error (interapplication manager)", "Bad occurrence", "Wait on unbound occurrence handler", "Occurrence queue overflow", "Datalog type conflict", "Unused", "Unrecognized type (interapplication manager)", "Memory corrupt", "Failed to make temporary DLL", "Old CIN version", "Drag socket not found", "Failed to load drop-object", "Failed to register OLE object", "Failed to release OLE object", "Format specifier type mismatch", "Unknown format specifier", "Too few format specifiers", "Too many format specifiers", "Scan failed", "Newer CIN version", "Error converting to variant", "Runtime menu error", "Password tampered", "Variant attribute not found", "Incompatible variant data type", "Event data is not available", "Event Store is not present", "Occurrence is not found", "Event Queue is not created", "Event info is not available", "Refnum passed is NULL", "Error retrieving Class GUID", "Error retrieving CoClass GUID", "Error retrieving TypeLib GUID.", "Bad built application magic bytes.", "Specific driver is different from the specific driver associated with the Logical Name.", "There is no session opened to the class driver.", "Max Error", "MAX - Error with config objects", "MAX - Error loading configuration", "MAX - Group not supported"]
        # "Current State"
        # "Do not delete, rename, or modify this frame.\n(this is used to capture unhandled states and typos)"
        # "Handle mistyped state name (developer tool)"
        n289 = Format Into String(format string="Software Exception: Unhandled State \"%s\"." ("message"), error in=w712, w707) -> (resulting string=w715:string, error out=w714:errorcluster)  [unwired: 1 in]
        n290 = call <vilib>:"Error Cluster From Error Code.vi"("show call chain? (False)"=TRUE, "error in (no error)"=w714, "error message (\"\")"=w715, "error code (0)"=w716) -> ("error out"=w713:errorcluster)  [unwired: 5 in]
        n291 = call <vilib>:"Add State(s) to Queue__JKI_lib_State_Machine.vi"("State(s) in (\"\")"=w711) -> ("States Out"=w710:string)  [unwired: 14 in]
      }
      frame "Initialize Core Data" {
        # "Do not delete, rename, or modify this frame.\n(this is used to determine panel behavior on exit)"
        # "originally closed?"
        # "exe?"
        # "If panel starts closed or is an EXE, then close it when we exit"
        n292 = property class="VI"() -> ("FP.State"=w721:T36)  [unwired: 2 in, 2 out]
        n293 = property class="App"() -> ("App.Kind"=w727:T37)  [unwired: 2 in, 2 out]
        n294 = control-ref of="Current VI Reference"() -> (w722:refnum<vi>)
        n295 = Equal?(x=w721, y=T36."Closed" ("Front Panel Window:State")) -> (x = y?=w719:bool)
        n296 = Equal?(x=w727, y=T37."Run Time System" ("Application:Kind")) -> (x = y?=w725:bool)
        n297 = Or(x=w719, y=w725) -> (x .or. y?=w723:bool)
        n298 = Bundle By Name(cluster=w724, "Core.Current VI Reference"=w722, "Core.Close Panel on Exit?"=w723) -> (w729:T39)
        n299 = call <vilib>:"Add State(s) to Queue__JKI_lib_State_Machine.vi"("State(s) in (\"\")"=w731) -> ("States Out"=w730:string)  [unwired: 14 in]
      }
      frame "Error Handler" {
        # "Unhandled Error -- Display it"
        # "Handle any errors here.\nYou can also output any states to clean-up after errors occur"
        # "Clear error"
        n300 = call <vilib>:"General Error Handler.vi"("error in (no error)"=w734) -> ()  [unwired: 10 in, 5 out]
        n301 = call <vilib>:"Add State(s) to Queue__JKI_lib_State_Machine.vi"("State(s) in Front (\"\")"="/* Post Error States", "State(s) in (\"\")"=w738) -> ("States Out"=w737:string)  [unwired: 13 in]
      }
      frame "Exit" {
        n302 = call <vilib>:"Add State(s) to Queue__JKI_lib_State_Machine.vi"("State(s) in (\"\")"=w744) -> ("States Out"=w743:string)  [unwired: 14 in]
      }
      frame "---------- Data ----------" {
        # "Do not put any code in this frame.\n(It is a separator no-op. You can make a copy of this frame to create a new Data frame)"
        n303 = call <vilib>:"Add State(s) to Queue__JKI_lib_State_Machine.vi"("State(s) in (\"\")"=w749) -> ("States Out"=w748:string)  [unwired: 14 in]
      }
      frame "Data: Initialize" {
        w756 = T40 {"Current VI Reference"=refnum, "Close Panel on Exit?"=FALSE}  # Core
        n304 = call "MessageAMC_Create.vi"("reference in"=refnum<class "MessageAMC.lvclass"> refnum, "error in (no error)"=w752, "message queue name"="GUI_DATA_VIEW") -> ("amc"=w751:refnum<class "MessageAMC.lvclass">, "error out"=w750:errorcluster)  [unwired: 15 in]
        n305 = Bundle("Core"=w756, "amc"=w751) -> (w757:T39)  [unwired: 1 in]
      }
      frame "Data: Cleanup" {
        # "Cleanup any data and references, here.\n(this is called automatically, by the Macro: Exit)"
        n306 = Unbundle By Name(w760) -> ("Core.Current VI Reference"=w763:refnum<vi>)
        n307 = Close Reference(reference=w763, error in (no error)=w762) -> (error out=w761:errorcluster)
        n308 = call <vilib>:"Add State(s) to Queue__JKI_lib_State_Machine.vi"("State(s) in (\"\")"=w765) -> ("States Out"=w764:string)  [unwired: 14 in]
      }
      frame "---------- Events ----------" {
        # "Do not put any code in this frame.\n(It is a separator no-op. You can make a copy of this frame to create a new UI frame)"
        n309 = call <vilib>:"Add State(s) to Queue__JKI_lib_State_Machine.vi"("State(s) in (\"\")"=w770) -> ("States Out"=w769:string)  [unwired: 14 in]
      }
      frame "Events: Register" {
        n310 = call "Read stop event.vi"("GUI in"=w772) -> ("stop event"=w771:refnum<user-event>)  [unwired: 8 in, 2 out]
        n311 = register-events(error in=w773, w771) -> (reference out=w775:refnum<event-registration>, error out=w774:errorcluster)  [unwired: 1 in]
      }
      frame "Events: Unregister" {
        # "Do not put any code in this frame.\n(It is a separator no-op. You can make a copy of this frame to create a new UI frame)"
        n312 = Unregister For Events(event registration refnum=w780, error in=w779) -> (error out=w778:errorcluster)
        n313 = call <vilib>:"Add State(s) to Queue__JKI_lib_State_Machine.vi"("State(s) in (\"\")"=w783) -> ("States Out"=w782:string)  [unwired: 14 in]
      }
      frame "---------- UI ----------" {
        # "Do not put any code in this frame.\n(It is a separator no-op. You can make a copy of this frame to create a new UI frame)"
        n314 = call <vilib>:"Add State(s) to Queue__JKI_lib_State_Machine.vi"("State(s) in (\"\")"=w788) -> ("States Out"=w787:string)  [unwired: 14 in]
      }
      frame "UI: Initialize" {
        "Multicolumn Listbox" <- -1 ("Multicolumn Listbox")
      }
      frame "UI: Cursor Set" {
        # "Argument"
        # "Set and Unset Cursor Busy.\n(Usage: \"UI: Cursor Set >> Busy|Idle\")"
        n315 = case shown="\"Idle\", Default" w795 {
          tunnel: w797 -> [w802 w804]
          tunnel: [w801 w803] -> w796
          frame "Idle", Default {
            n316 = call <vilib>:"Unset Busy.vi"("error in (no error)"=w802) -> ("error out"=w801:errorcluster)  [unwired: 10 in]
          }
          frame "Busy" {
            n317 = call <vilib>:"Set Busy.vi"("error in (no error)"=w804) -> ("error out"=w803:errorcluster)  [unwired: 9 in, 1 out]
          }
        }
        n318 = call <vilib>:"Add State(s) to Queue__JKI_lib_State_Machine.vi"("State(s) in (\"\")"=w800) -> ("States Out"=w799:string)  [unwired: 14 in]
      }
      frame "UI: Front Panel State" {
        # "Argument"
        # "Set Front Panel Open or Closed\n(Usage: \"UI: Front Panel State >> Open|Close\")"
        n319 = Unbundle By Name(w808) -> ("Core.Current VI Reference"=w807:refnum<vi>)
        n320 = case shown="\"Minimize\", \"Minimized\"" w806 {
          tunnel: w810 -> [w818 w833 w844 w857 w870]
          tunnel: [w820 w834 w846 w859 w872] -> w809
          tunnel: w807 -> [w819 w831 w845 w858 w871]
          frame "Open", "Standard", Default {
            w813 = T36."Standard" ("State")
            n321 = property class="VI"(reference=w819, error in=w818) -> (reference out=w816:refnum<vi>, error out=w817:errorcluster, "FP.State"=w815:T36)
            n322 = Not Equal?(x=w815, y=w813) -> (x != y?=w814:bool)
            n323 = case shown="True" w814 {
              tunnel: [w824 w826] -> w820
              tunnel: w817 -> [w823 w826]
              tunnel: w816 -> [w822 _]
              tunnel: w813 -> [w821 _]
              frame True {
                n324 = invoke class="VI" method="FP.Open"(reference=w822, error in=w823, "Activate"=TRUE, "State"=w821) -> (error out=w824:errorcluster)  [unwired: 1 in, 4 out]
              }
              frame False {
              }
            }
          }
          frame "Close", "Closed" {
            n325 = property class="VI"(reference=w831, error in=w833) -> (reference out=w830:refnum<vi>, error out=w832:errorcluster, "FP.State"=w828:T36)
            n326 = Not Equal?(x=w828, y=T36."Closed" ("Front Panel Window:State")) -> (x != y?=w827:bool)
            n327 = case shown="True" w827 {
              tunnel: [w835 w838] -> w834
              tunnel: w832 -> [w835 w837]
              tunnel: w830 -> [_ w836]
              frame False {
              }
              frame True {
                n328 = invoke class="VI" method="FP.Close"(reference=w836, error in=w837) -> (error out=w838:errorcluster)  [unwired: 1 in, 2 out]
              }
            }
          }
          frame "Hidden", "Hide" {
            w839 = T36."Hidden" ("State")
            n329 = property class="VI"(reference=w845, error in=w844) -> (reference out=w842:refnum<vi>, error out=w843:errorcluster, "FP.State"=w841:T36)
            n330 = Not Equal?(x=w841, y=w839) -> (x != y?=w840:bool)
            n331 = case shown="True" w840 {
              tunnel: [w850 w851] -> w846
              tunnel: w843 -> [w849 w851]
              tunnel: w842 -> [w848 _]
              tunnel: w839 -> [w847 _]
              frame True {
                n332 = invoke class="VI" method="FP.Open"(reference=w848, error in=w849, "State"=w847) -> (error out=w850:errorcluster)  [unwired: 2 in, 4 out]
              }
              frame False {
              }
            }
          }
          frame "Minimize", "Minimized" {
            w852 = T36."Minimized" ("State")
            n333 = property class="VI"(reference=w858, error in=w857) -> (reference out=w855:refnum<vi>, error out=w856:errorcluster, "FP.State"=w854:T36)
            n334 = Not Equal?(x=w854, y=w852) -> (x != y?=w853:bool)
            n335 = case shown="True" w853 {
              tunnel: [w863 w864] -> w859
              tunnel: w856 -> [w862 w864]
              tunnel: w855 -> [w861 _]
              tunnel: w852 -> [w860 _]
              frame True {
                n336 = invoke class="VI" method="FP.Open"(reference=w861, error in=w862, "State"=w860) -> (error out=w863:errorcluster)  [unwired: 2 in, 4 out]
              }
              frame False {
              }
            }
          }
          frame "Maximize", "Maximized" {
            w865 = T36."Maximized" ("State")
            n337 = property class="VI"(reference=w871, error in=w870) -> (reference out=w868:refnum<vi>, error out=w869:errorcluster, "FP.State"=w867:T36)
            n338 = Not Equal?(x=w867, y=w865) -> (x != y?=w866:bool)
            n339 = case shown="True" w866 {
              tunnel: [w876 w877] -> w872
              tunnel: w869 -> [w875 w877]
              tunnel: w868 -> [w874 _]
              tunnel: w865 -> [w873 _]
              frame True {
                n340 = invoke class="VI" method="FP.Open"(reference=w874, error in=w875, "State"=w873) -> (error out=w876:errorcluster)  [unwired: 2 in, 4 out]
              }
              frame False {
              }
            }
          }
        }
        n341 = call <vilib>:"Add State(s) to Queue__JKI_lib_State_Machine.vi"("State(s) in (\"\")"=w812) -> ("States Out"=w811:string)  [unwired: 14 in]
      }
      frame "---------- Macro ----------" {
        # "Do not put any code in this frame.\n(It is a separator no-op. You can make a copy of this frame to create a new Macro frame)"
        n342 = call <vilib>:"Add State(s) to Queue__JKI_lib_State_Machine.vi"("State(s) in (\"\")"=w882) -> ("States Out"=w881:string)  [unwired: 14 in]
      }
      frame "Macro: Initialize" {
        n343 = call <vilib>:"Add State(s) to Queue__JKI_lib_State_Machine.vi"("State(s) in Front (\"\")"="Data: Initialize\nInitialize Core Data\nEvents: Register\nUI: Initialize\n// UI: Front Panel State >> Open\n\n\nAction: Read Config\nAction: Update Indicators\n", "State(s) in (\"\")"=w888) -> ("States Out"=w887:string)  [unwired: 13 in]
      }
      frame "Macro: Update" {
        n344 = call <vilib>:"Add State(s) to Queue__JKI_lib_State_Machine.vi"("State(s) in Front (\"\")"="Action: Update Indicators\nAction: Write Config", "State(s) in (\"\")"=w894) -> ("States Out"=w893:string)  [unwired: 13 in]
      }
      frame "Macro: Exit" {
        # "Exit Macro\n(This is called once, when the VI exits)"
        n345 = Unbundle By Name(w903) -> ("Core.Close Panel on Exit?"=w902:bool)
        n346 = Select(t="UI: Front Panel State >> Close", s=w902, f="") -> (s? t:f=w899:string)
        n347 = call <vilib>:"Add State(s) to Queue__JKI_lib_State_Machine.vi"("State(s) in Front (\"\")"="Action: Write Config", "State(s) in (\"\")"=w899, "State(s) at Back (\"\")"="Data: Cleanup\nEvents: Unregister\nExit") -> ("States Out"=w897:string)  [unwired: 12 in]
        n348 = call <vilib>:"Add State(s) to Queue__JKI_lib_State_Machine.vi"("State(s) in Front (\"\")"=w897, "State(s) in (\"\")"=w906) -> ("States Out"=w905:string)  [unwired: 13 in]
      }
      frame "---------- Action ----------" {
      }
      frame "Action: Read Config" {
      }
      frame "Action: Write Config" {
      }
      frame "Action: Update Indicators" {
      }
      frame "Action: Update Channels TBL" {
      }
    }
  }
  n349 = flat-sequence {
    frame #0 {
    }
    frame #1 {
    }
  }
  n350 = flat-sequence {
    tunnel: w7 -> [w928]
    frame #0 {
      n351 = local write "stop"(TRUE ("stop")) -> ()
      "error out" <- w928
    }
  }
